vi "ExperimentCode_nodaq.vi"() -> ()   [LabVIEW 2017]
uses:
  <vilib>/Analysis/baseanly.llb/Mean (DBL).vi
  <vilib>/Instr/_visa.llb/VISA Configure Serial Port (Instr).vi
  <vilib>/express/express shared/transition.llb/Dynamic To Waveform Array.vi
  <vilib>/express/express signal manip/GetorSetDDTAttributes/Set DDT Attributes/SetT0.vi
  <vilib>/express/express shared/transition.llb/Waveform Array To Dynamic.vi
  <vilib>/express/express signal manip/GetorSetDDTAttributes/Set DDT Attributes/Set DDT Properties.xnode
  <vilib>/Analysis/NI_AALPro.lvlib
  <vilib>/Analysis/NI_AALBase.lvlib
panel:
  in  "Tab Control":enum32{"Setup ", "Experiment Controls", "Debug"}(tab)=enum."Experiment Controls"
  in  "Axial Force Slope":dbl=1.0
  in  "Axial Force Intercept":dbl
  in  "Side Force Slope":dbl=1.0
  in  "Side Force Intercept":dbl
  in  "Yaw Moment Slope":dbl=1.0
  in  "Yaw Moment Intercept":dbl
  in  "Max Torque":dbl=21.3
  in  "Servo 1 Zero Offset":dbl
  in  "Servo 2 Zero Offset":dbl
  in  "Servo 3 Zero Offset":dbl
  in  "Servo 4 Zero Offset":dbl
  in  "Servo 5 Zero Offset":dbl
  in  "Servo 5 Torque Intercept":dbl
  in  "Servo 5 Torque Slope":dbl=1.0
  in  "Servo 5 Position Intercept":dbl
  in  "Servo 5 Position Slope":dbl=1.0
  in  "Servo 4 Torque Intercept":dbl
  in  "Servo 4 Torque Slope":dbl=1.0
  in  "Servo 4 Position Intercept":dbl
  in  "Servo 4 Position Slope":dbl=1.0
  in  "Servo 3 Torque Intercept":dbl
  in  "Servo 3 Torque Slope":dbl=1.0
  in  "Servo 3 Position Intercept":dbl=-111.82
  in  "Servo 3 Position Slope":dbl=0.00449
  in  "Servo 2 Torque Intercept":dbl
  in  "Servo 2 Torque Slope":dbl=1.0
  in  "Servo 2 Position Intercept":dbl=-97.9723
  in  "Servo 2 Position Slope":dbl=0.00488
  in  "Servo 1 Torque Intercept":dbl
  in  "Servo 1 Torque Slope":dbl=1.0
  in  "Servo 1 Position Intercept":dbl=-99.625
  in  "Servo 1 Position Slope":dbl=0.004988
  in  "Plot Last x Seconds":dbl=60.0
  in  "COM Port":refnum<visa-resource-name>
  in  "Buad Rate":i32(ring)=115200 items=["2400"=2400, "4800"=4800, "9600"=9600, "14400"=14400, "19200"=19200, "28800"=28800, "38400"=38400, "57600"=57600, "115200"=115200]
  in  "Lowest Servo Angle":dbl=-65.0
  in  "Highest Servo Angle":dbl=65.0
  in  "Number of Servos":dbl=5.0
  out "Lift FFT":cluster{"timeout (s)":dbl, dbl, dbl[]}(graph)={"timeout (s)"=0.0, 0.12149192078726764, [0.041647829769514415, 0.5815679381268424, 0.2410963163674246, 0.13249316216492138, 0.09139863383267581, 0.06777994108166811, 0.05676278057361634, 0.046891488943555756, 0.04170299677912171, 0.03813645823405653, 0.032751623310567676, 0.03235242616779546, 0.02857646287326414, 0.027921332836055062, 0.026075669248962027, 0.025506839186418245, 0.02300088021285802, 0.022263519164960176, 0.020785068115577936, 0.020572576904436635, 0.019706083690027066, 0.01933094658327721, 0.018088168860478246, 0.018107278585544298, 0.016955162903130913, 0.016878745360566313, 0.015869739803903514, 0.015674152094024396, 0.016464851454026343, 0.015714406087046065, 0.015341040986334412, 0.015154899432712336, 0.014786629089704205, 0.01448548753300844, 0.014186097789199267, 0.014076976739574329, 0.013620814630327938, 0.014015320026164364, 0.013807357325215744, 0.01339057225347958, 0.01298234875346484, 0.013354575711390817, 0.013214518458269849, 0.013075613311439785, 0.012989188265392547, 0.012875952831802175]}
  out "Maximum Torque Exceeded":bool
  in  "Amplitude (deg)":dbl=3.0
  in  "Save":bool
  in  "Stop VI":bool
  in  "Sample Frequency":dbl=100.0 step=50.0
  out "Servo Torque":cluster{" Time Offset":dbl, dbl, dbl[][]}(graph)
  in  "Amplitude (cm)":dbl=4.0
  in  "Length of Segments":dbl=10.0
  in  "Number of Waves":dbl=1.0
  in  "Wave Exponential":dbl=2.0
  in  "Frequency":dbl=1.0
  in  "Wave Form":u16(ring) items=["Sine", "Exponentional Sine", "Second Mode Bending", "Flat Plate"]
  in  "Wind Up Waveform":bool
  in  "Mode 1 Amplitude":dbl=0.1 step=0.1
  in  "Mode 2 Amplitude":dbl=0.2 step=0.1
  in  "Mode 1 Phase":dbl step=0.1
  in  "Mode 2 Phase":dbl=0.8499 step=0.1
  in  "Wind Down Waveform":bool
  in  "Wind Down Time":i32=5
  out "Waveform":cluster{"X Nodes":dbl[], "Y Nodes":dbl[]}[](graph)
  in  "Servo Input":bool
  in  "Send To Waveform to MBE":bool
  in  "Servo 5 Input":dbl
  in  "Servo 4 Input":dbl
  in  "Servo 3 Input":dbl
  in  "Servo 2 Input":dbl
  in  "Servo 1  Input":dbl
  out "Force and Moment Data":cluster{" Time Offset":dbl, "mean":dbl, dbl[][]}(graph)
  out "Minimum or Maximum Angle Exceeded":bool
  in  "Filename":path=path "test.tdms"
  out "Drag FFT":cluster{"timeout (s)":dbl, dbl, dbl[]}(graph)={"timeout (s)"=0.0, 0.12149192078726764, [0.08329565953902883, 1.1631358762536848, 0.4821926327348492, 0.26498632432984276, 0.18279726766535162, 0.13555988216333623, 0.11352556114723268, 0.09378297788711151, 0.08340599355824342, 0.07627291646811306, 0.06550324662113535, 0.06470485233559092, 0.05715292574652828, 0.055842665672110124, 0.052151338497924055, 0.05101367837283649, 0.04600176042571604, 0.04452703832992035, 0.04157013623115587, 0.04114515380887327, 0.03941216738005413, 0.03866189316655442, 0.03617633772095649, 0.036214557171088596, 0.033910325806261826, 0.03375749072113263, 0.03173947960780703, 0.03134830418804879, 0.03292970290805269, 0.03142881217409213, 0.030682081972668824, 0.030309798865424672, 0.02957325817940841, 0.02897097506601688, 0.028372195578398533, 0.028153953479148657, 0.027241629260655875, 0.028030640052328727, 0.02761471465043149, 0.02678114450695916, 0.02596469750692968, 0.026709151422781633, 0.026429036916539698, 0.02615122662287957, 0.025978376530785094, 0.02575190566360435]}
  in  "Comment":string
  out "Yaw FFT":cluster{"timeout (s)":dbl, dbl, dbl[]}(graph)={"timeout (s)"=0.0, 0.12149192078726764, [0.004164782976951441, 0.05815679381268424, 0.024109631636742457, 0.013249316216492139, 0.009139863383267582, 0.006777994108166813, 0.005676278057361634, 0.004689148894355577, 0.0041702996779121706, 0.0038136458234056527, 0.0032751623310567674, 0.0032352426167795464, 0.0028576462873264145, 0.0027921332836055067, 0.0026075669248962034, 0.002550683918641824, 0.002300088021285804, 0.002226351916496017, 0.0020785068115577923, 0.0020572576904436613, 0.0019706083690027043, 0.0019330946583277187, 0.0018088168860478228, 0.001810727858554431, 0.0016955162903130908, 0.0016878745360566349, 0.001586973980390353, 0.0015674152094024417, 0.001646485145402633, 0.0015714406087046053, 0.00153410409863344, 0.0015154899432712331, 0.0014786629089704193, 0.001448548753300844, 0.001418609778919927, 0.0014076976739574325, 0.0013620814630327948, 0.0014015320026164368, 0.0013807357325215724, 0.0013390572253479574, 0.0012982348753464844, 0.001335457571139084, 0.0013214518458269826, 0.0013075613311439762, 0.0012989188265392561, 0.0012875952831802166]}
  out "Specified Time Delay":dbl
  out "Calculated Time Delay":dbl
  out "Time Elapsed":dbl
  out "Output Angles":dbl[](array[numeric])
  out "Input Angles":dbl[](array[numeric])
  out "Pos5 number":dbl
  out "Pos4 number":dbl
  out "Pos3 number":dbl
  out "Pos2 number":dbl
  out "Pos1 number":dbl
  out "Torq1 number":dbl
  out "Torq2 number":dbl
  out "Torq3 number":dbl
  out "Torq4 number":dbl
  out "Torq5 number":dbl
  out "Servo 1 Position":cluster{" Time Offset":dbl, "mean":dbl, dbl[][]}(graph)
  out "Servo 2 Position":cluster{" Time Offset":dbl, "mean":dbl, dbl[][]}(graph)
  out "Servo 3 Position":cluster{" Time Offset":dbl, "mean":dbl, dbl[][]}(graph)
  out "Servo 4 Position":cluster{" Time Offset":dbl, "mean":dbl, dbl[][]}(graph)
  out "Servo 5 Position":cluster{" Time Offset":dbl, "mean":dbl, dbl[][]}(graph)
  out "Sent to Arduino":string
  out "Bytes at port":cluster{i32, dbl, dbl[]}(graph)
  out "Read Buffer":string
  out "X Nodes":dbl[](array[numeric])
  out "Y Nodes":dbl[](array[numeric])
  # "deg"
  # "deg"
  # "deg"
  # "deg"
  # "deg"
  # "Waveform"
  # "Manual"
  # "cm"
  # "Hz"
  # "Off"
  # "On"
  # "rad"
  # "rad"
  # "Off"
  # "On"
  # "Hz"
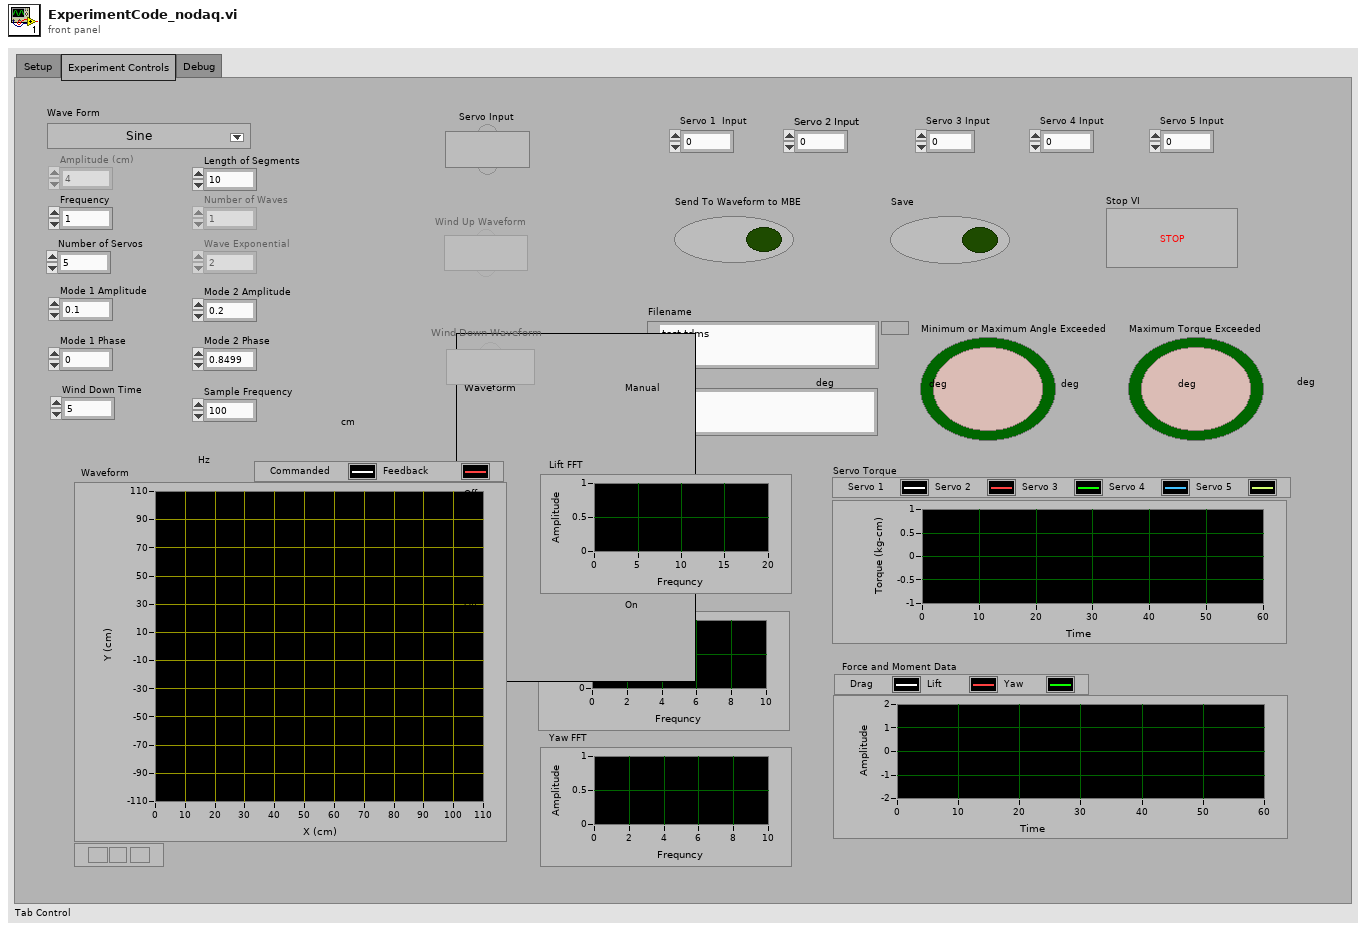
[diagram p1: front panel]
types:
  T1 = enum8{"Enabled", "Disabled", "Disabled and Grayed Out"}
  T2 = cluster{"Amplitude (deg)":dbl, "Amplitude (cm)":dbl, "Frequency":dbl, "Number of Waves":dbl, "Length of Segments":dbl, "Wave Exponential":dbl, "Number of Servos":dbl, "Mode 1 Amplitude":dbl, "Mode 2 Amplitude":dbl, "Mode 1 Phase":dbl, "Mode 2 Phase":dbl}
  T3 = cluster{"timeout (s)":dbl, "df":dbl, "Amp Spectrum Mag (Vrms)":dbl[]}
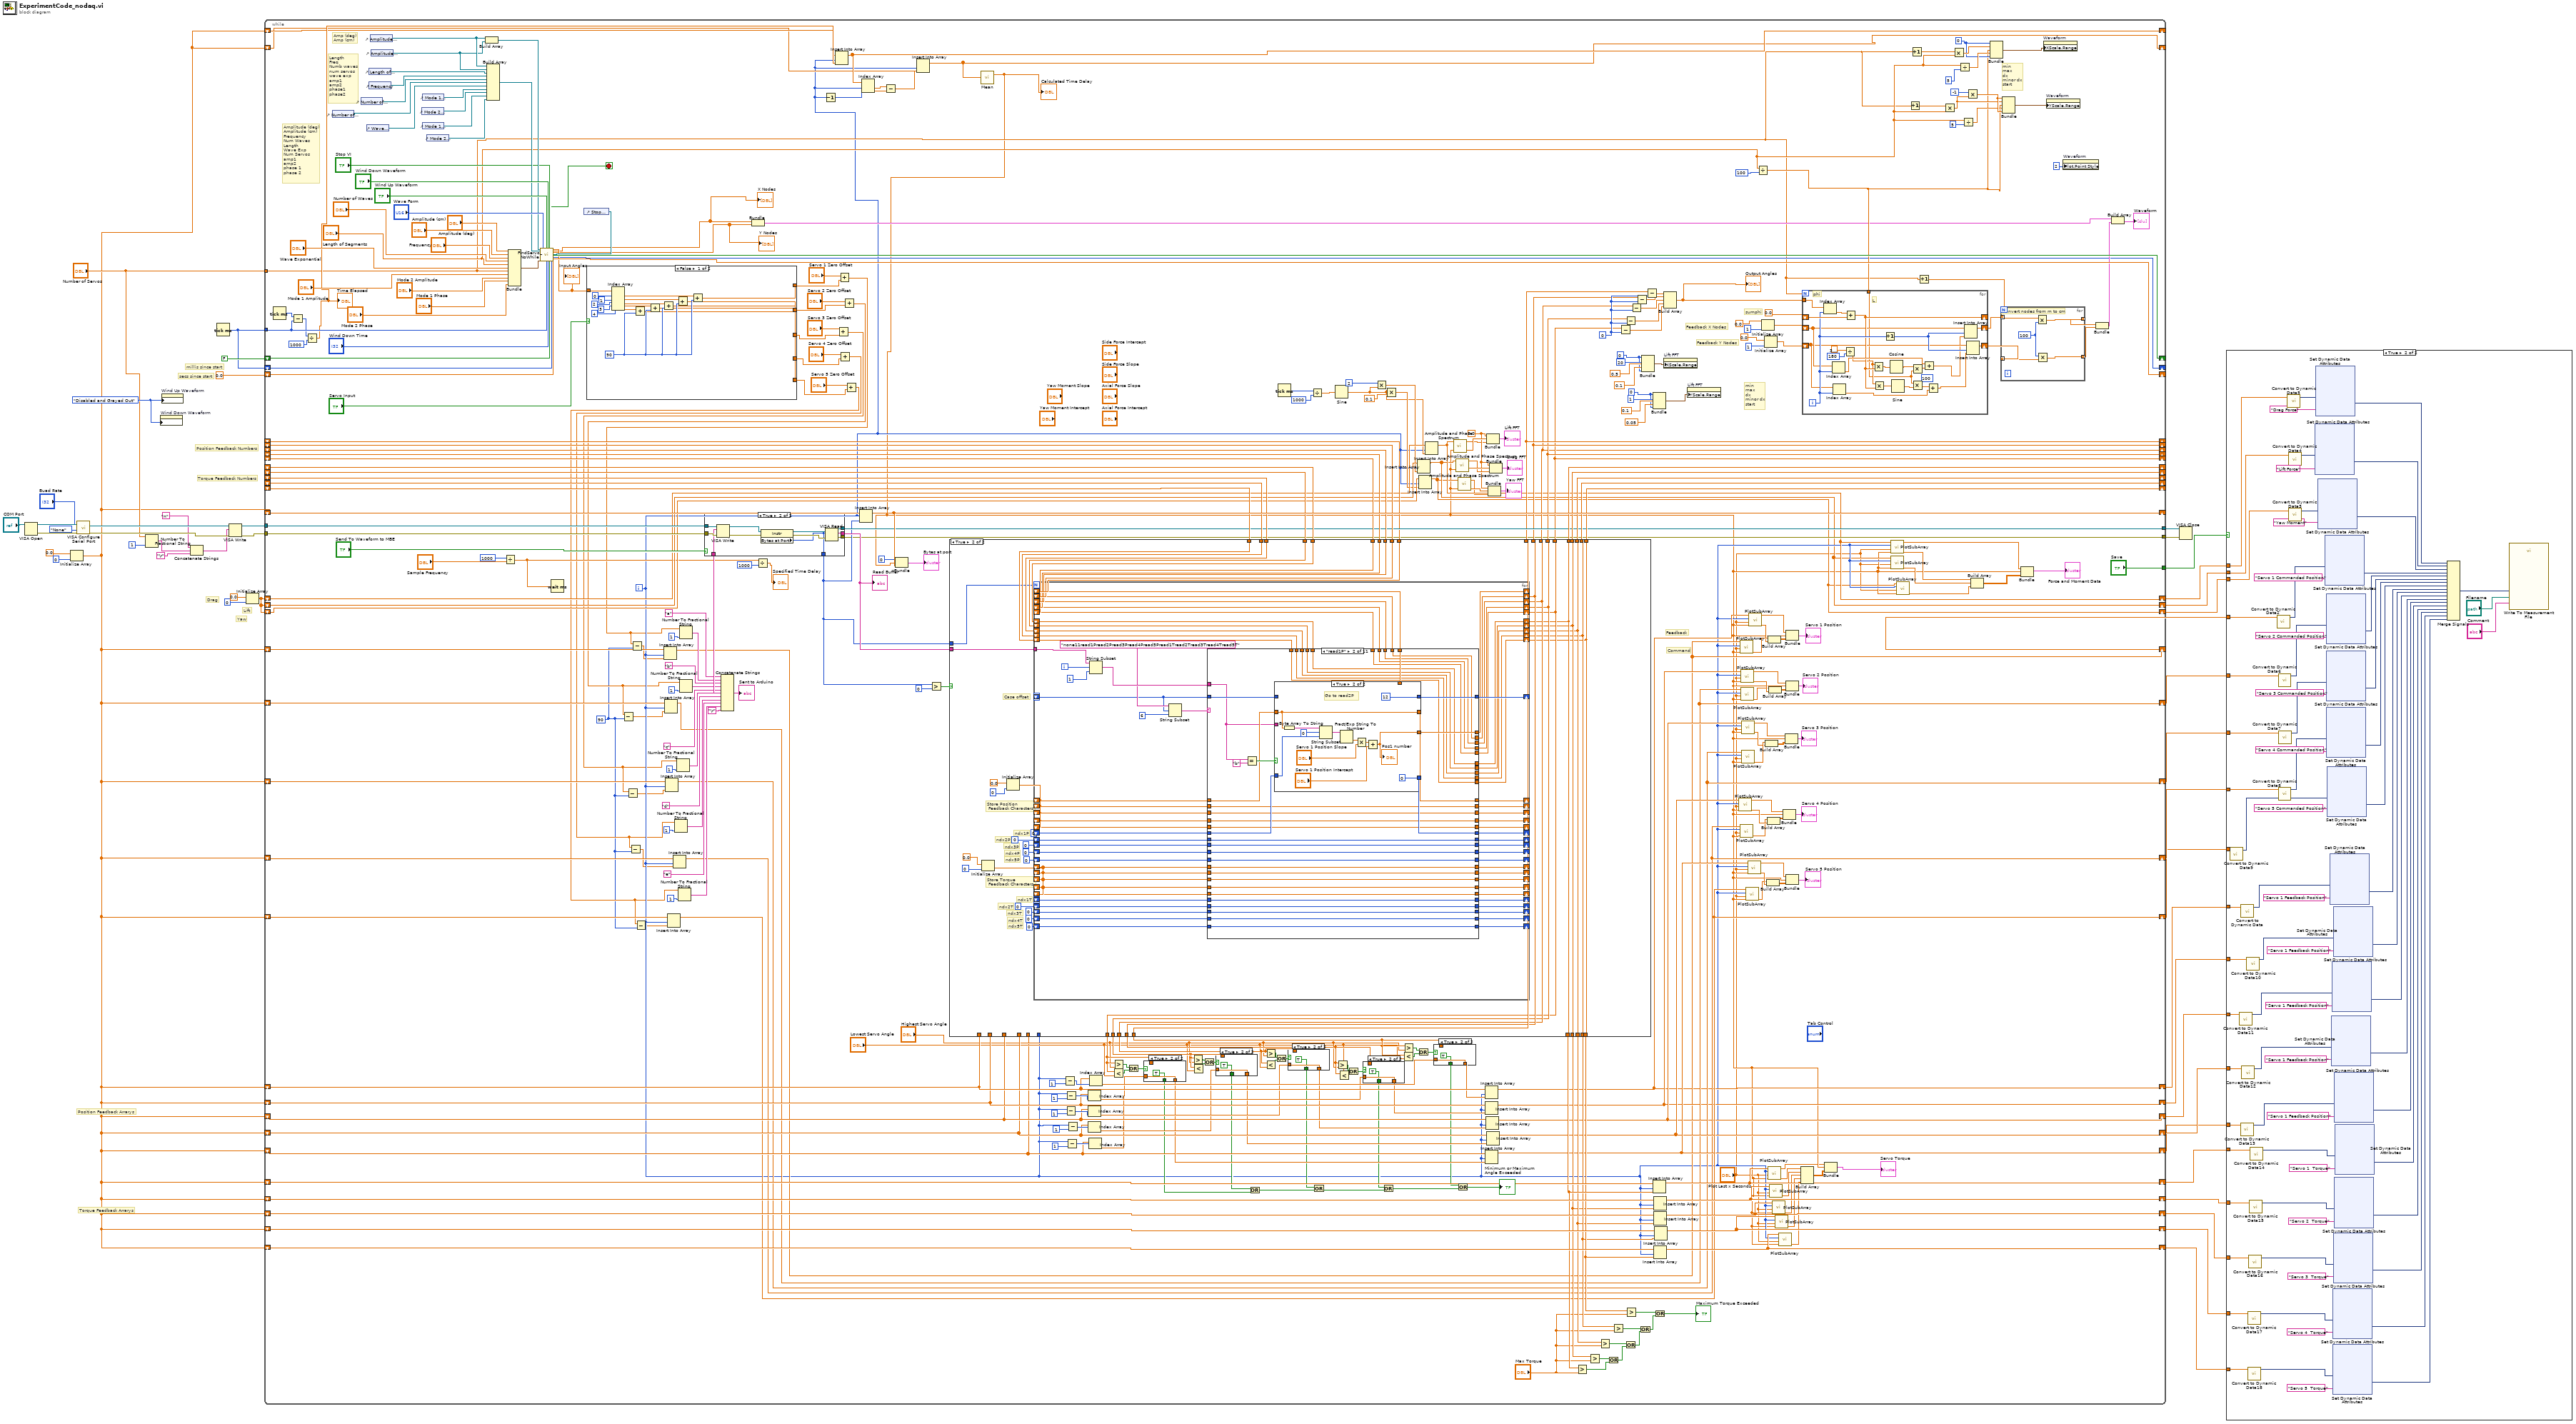
[diagram p0: block diagram]
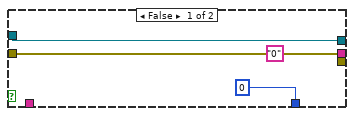
[diagram p3: hidden frame]
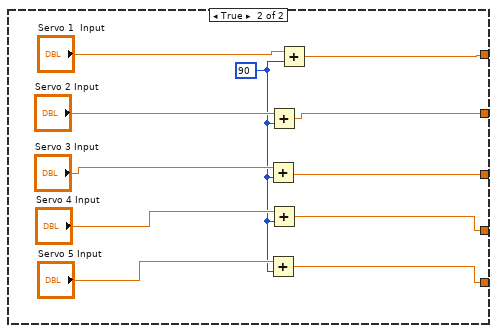
[diagram p4: hidden frame]
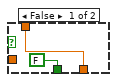
[diagram p5: hidden frame]
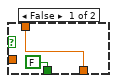
[diagram p6: hidden frame]
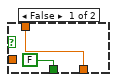
[diagram p7: hidden frame]
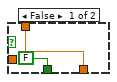
[diagram p8: hidden frame]
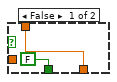
[diagram p9: hidden frame]
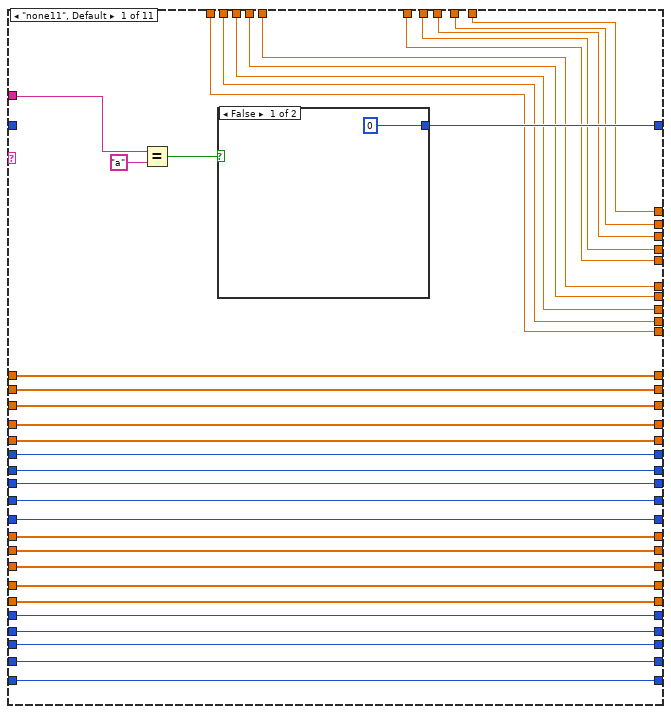
[diagram p11: hidden frame]
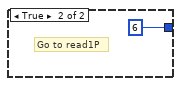
[diagram p12: hidden frame]
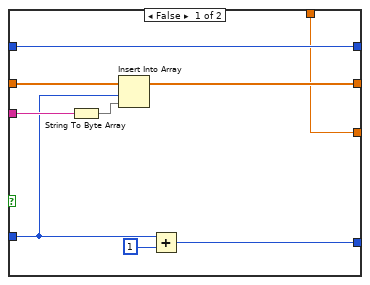
[diagram p13: hidden frame]
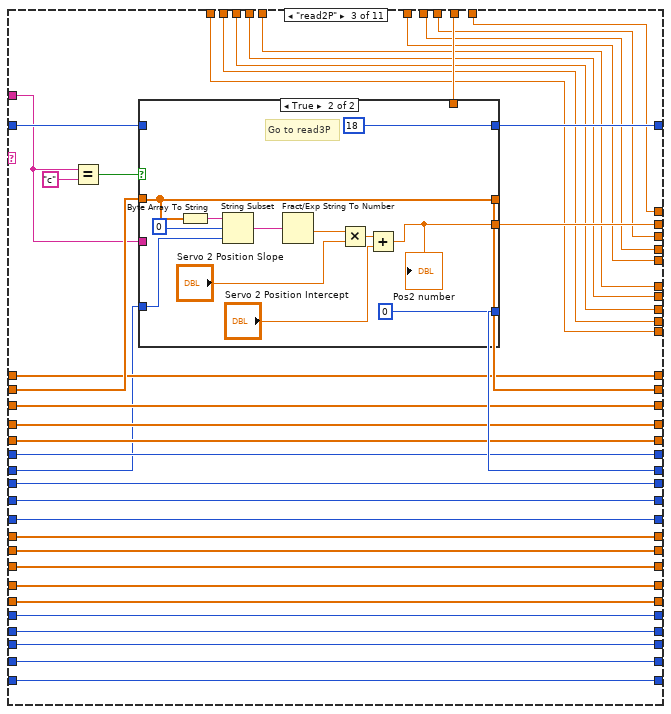
[diagram p14: hidden frame]
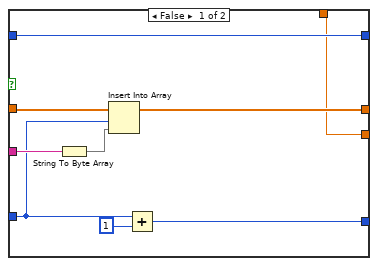
[diagram p15: hidden frame]
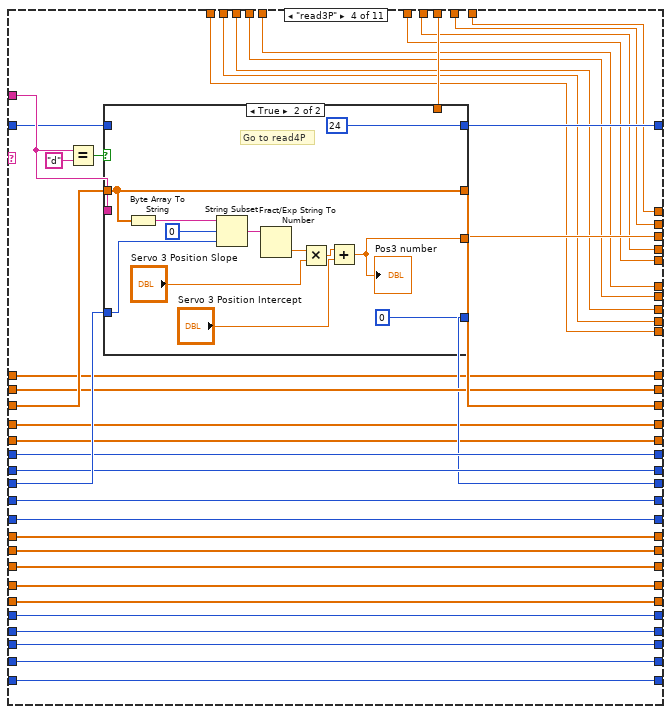
[diagram p16: hidden frame]
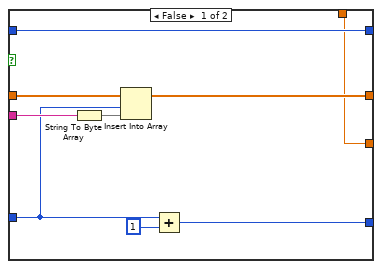
[diagram p17: hidden frame]
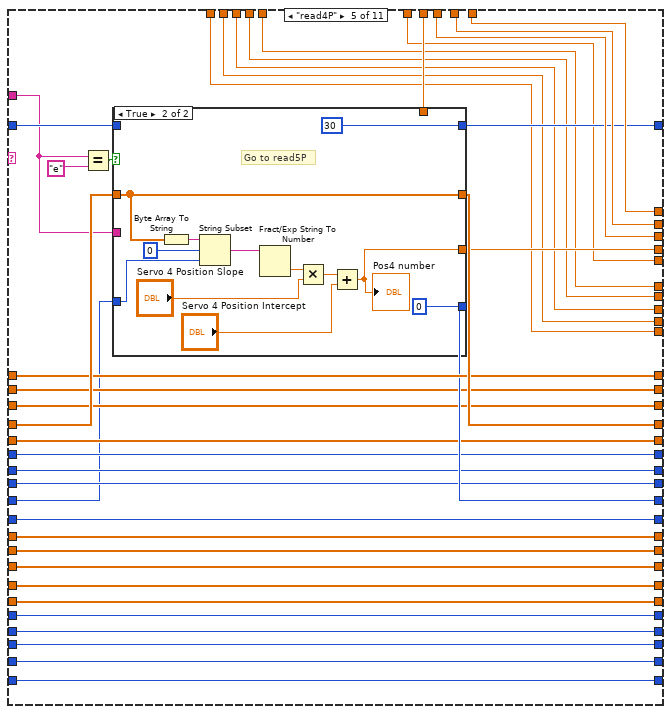
[diagram p18: hidden frame]
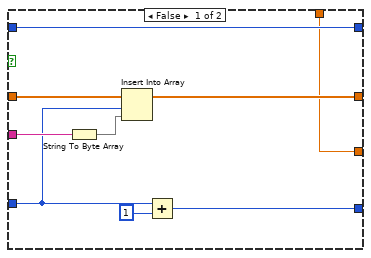
[diagram p19: hidden frame]
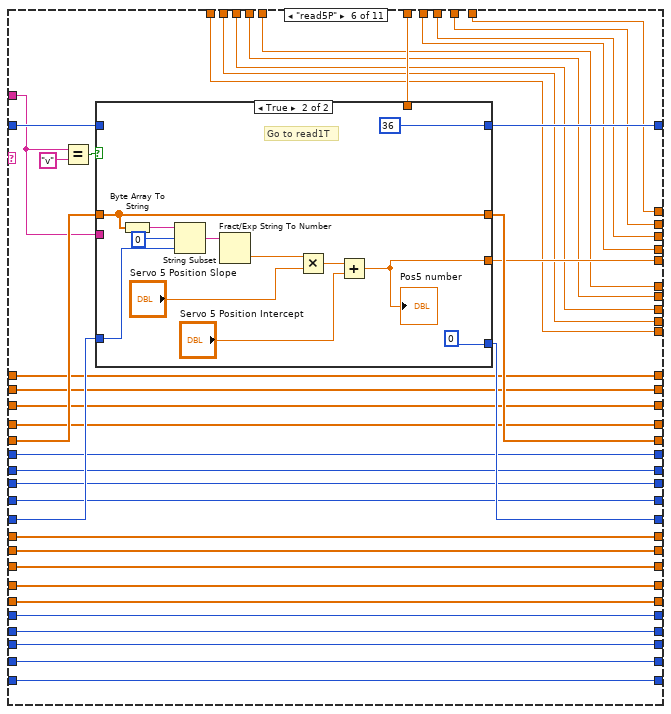
[diagram p20: hidden frame]
diagram:
  w28 = T1."Disabled and Grayed Out" ("Disabled")
  # "Yaw"
  # "Lift"
  # "secs since start"
  # "millis since start"
  # "Drag"
  # "Torque Feedback Numbers"
  # "Position Feedback Numbers"
  # "Torque Feedback Arrarys"
  # "Position Feedback Arrarys"
  n1 = VISA Open(VISA resource name="COM Port") -> (VISA resource name=w43:refnum<visa-resource-name>, error out=w41:errorcluster)  [unwired: 4 in]
  n2 = Initialize Array(0.0 ("element"), 0 ("dimension size")) -> (w1:dbl[])
  n3 = call-poly "VISA Configure Serial Port"("VISA resource name"=w43, "baud rate (9600)"="Buad Rate", "parity (0:none)"=enum16{"None", "Odd", "Even", "Mark", "Space"}."None", "error in (no error)"=w41) -> ("VISA resource name out"=w11:refnum<visa-resource-name>, "error out"=w10:errorcluster)  [unwired: 10 in]
  n4 = Number To Fractional String(number="Number of Servos", precision (6)=1) -> (F-format string=w6:string)  [unwired: 2 in]
  n5 = property on="Wind Down Waveform" class="Bool (strict)"("DisabledEnum"=w28) -> ()  [unwired: 2 in, 2 out]
  n6 = property on="Wind Up Waveform" class="Bool (strict)"("DisabledEnum"=w28) -> ()  [unwired: 2 in, 2 out]
  n7 = Concatenate Strings("n", w6, "\r") -> (w2:string)
  n8 = Tick Count (ms)() -> (millisecond timer value=w37:u32)
  n9 = VISA Write(VISA resource name=w11, write buffer=w2, error in (no error)=w10) -> (VISA resource name out=w9:refnum<visa-resource-name>, error out=w8:errorcluster)  [unwired: 1 out]
  n10 = Initialize Array(0.0 ("element"), 0 ("dimension size")) -> (w29:dbl[])
  n11 = while {
    shift-right: [w387] -> _
    shift-left: w1 -> [w388]
    shift-right: [w93] -> w35
    shift-left: w1 -> [w364]
    shift-right: [w95] -> w24
    shift-left: w1 -> [w363]
    shift-right: [w99] -> w23
    shift-left: w1 -> [w362]
    shift-right: [w101] -> w22
    shift-left: w1 -> [w361]
    shift-right: [w109] -> w21
    shift-left: w1 -> [w360]
    shift-right: [w92] -> w31
    shift-left: w1 -> [w328]
    shift-right: [w94] -> w20
    shift-left: w1 -> [w320]
    shift-right: [w98] -> w19
    shift-left: w1 -> [w317]
    shift-right: [w102] -> w18
    shift-left: w1 -> [w314]
    shift-right: [w108] -> w17
    shift-left: w1 -> [w284]
    shift-right: [w185] -> _
    shift-left: _ -> [w331]
    shift-right: [w184] -> _
    shift-left: _ -> [w350]
    shift-right: [w181] -> _
    shift-left: _ -> [w353]
    shift-right: [w183] -> _
    shift-left: _ -> [w352]
    shift-right: [w182] -> _
    shift-left: _ -> [w351]
    shift-right: [w344] -> _
    shift-left: _ -> [w345]
    shift-right: [w343] -> _
    shift-left: _ -> [w346]
    shift-right: [w342] -> _
    shift-left: _ -> [w347]
    shift-right: [w341] -> _
    shift-left: _ -> [w348]
    shift-right: [w340] -> _
    shift-left: _ -> [w349]
    shift-right: [w226] -> w16
    shift-left: w1 -> [w339]
    shift-right: [w224] -> w15
    shift-left: w1 -> [w338]
    shift-right: [w223] -> w14
    shift-left: w1 -> [w337]
    shift-right: [w222] -> w13
    shift-left: w1 -> [w336]
    shift-right: [w225] -> w12
    shift-left: w1 -> [w335]
    tunnel: w8 -> [w283]
    shift-right: [w89] -> w27
    shift-left: w29 -> [w147]
    tunnel: w37 -> [w126]
    shift-right: [w277] -> _
    shift-left: FALSE -> [w274]
    shift-right: [w116] -> _
    shift-left: w37 -> [w122]
    shift-right: [w276] -> _
    shift-left: 0.0 ("S since stop Shift Out") -> [w123]
    tunnel: ["Save"] -> w34
    tunnel: w9 -> [w282]
    tunnel: [w332] -> w33
    tunnel: [w154] -> w32
    shift-right: [w73] -> w26
    shift-left: w29 -> [w146]
    shift-right: [w72] -> w25
    shift-left: w29 -> [w145]
    shift-right: [w113] -> _
    shift-left: w1 -> [w120]
    tunnel: "Number of Servos" -> [w115]
    shift-right: [w110] -> _
    shift-left: w1 -> [w111]
    i -> [w84]
    stop <- w236 stop-if-true
    w49 = 90
    w132 = 0
    w136 = 0
    w65 = 0.0 ("timeout (s)")
    w170 = 0
    w186 = 0
    # "min\nmax\ndx\nminor dx\nstart"
    # "min\nmax\ndx\nminor dx\nstart"
    # "Feedback Y Nodes"
    # "Feedback X Nodes"
    # "sumphi"
    # "Command"
    # "Feedback"
    # "Amplitude (deg)\nAmplitude (cm)\nFrequency\nNum Waves\nLength\nWave Exp\nNum Servos\namp1\namp2\nphase 1\nphase 2"
    # "Amp (deg)\nAmp (cm)"
    # "Length\nFreq\nNumb waves\nnum servos\nwave exp\namp1\namp2\nphase1\nphase2"
    n12 = Tick Count (ms)() -> (millisecond timer value=w127:u32)
    n13 = Subtract(x=w127, y=w126) -> (x-y=w125:u32)
    n14 = Divide(x=w125, y=1000) -> (x/y=w121:dbl)
    "Time Elapsed" <- w121
    n15 = control-ref of="Number of Servos"() -> (w114:refnum<vi>)
    n16 = control-ref of="Number of Waves"() -> (w259:refnum<vi>)
    n17 = control-ref of="Wave Exponential"() -> (w258:refnum<vi>)
    n18 = control-ref of="Length of Segments"() -> (w261:refnum<vi>)
    n19 = control-ref of="Frequency"() -> (w260:refnum<vi>)
    n20 = control-ref of="Amplitude (deg)"() -> (w241:refnum<vi>)
    n21 = control-ref of="Amplitude (cm)"() -> (w240:refnum<vi>)
    n22 = control-ref of="Mode 2 Amplitude"() -> (w256:refnum<vi>)
    n23 = control-ref of="Mode 1 Amplitude"() -> (w257:refnum<vi>)
    n24 = control-ref of="Mode 1 Phase"() -> (w255:refnum<vi>)
    n25 = control-ref of="Mode 2 Phase"() -> (w254:refnum<vi>)
    n26 = Build Array(w241, w240) -> (w243:refnum<vi>[])
    n27 = Build Array(w241, w240, w261, w260, w259, w114, w258, w257, w256, w255, w254) -> (w242:refnum<vi>[])
    n28 = Divide(x=1000, y="Sample Frequency") -> (x/y=w129:dbl)
    n29 = Bundle("Amplitude (deg)"="Amplitude (deg)", "Amplitude (cm)"="Amplitude (cm)", "Frequency"="Frequency", "Number of Waves"="Number of Waves", "Length of Segments"="Length of Segments", "Wave Exponential"="Wave Exponential", "Number of Servos"=w115, "Mode 1 Amplitude"="Mode 1 Amplitude", "Mode 2 Amplitude"="Mode 2 Amplitude", "Mode 1 Phase"="Mode 1 Phase", "Mode 2 Phase"="Mode 2 Phase") -> (w244:T2)  [unwired: 1 in]
    n30 = Wait (ms)(milliseconds to wait=w129) -> ()  [unwired: 1 out]
    n31 = control-ref of="Stop Reference"() -> (w273:refnum<vi>)
    n32 = call "FindServo_NoWhile.vi"("Amplitude Reference Array"=w243, "Parameter Reference Arrary"=w242, "Parameter Cluster"=w244, "Wave Form"="Wave Form", "Wind Up"="Wind Up Waveform", "Start Time (Tick Count-millis)"=w126, "Wind Down"="Wind Down Waveform", "Wind Down Time"="Wind Down Time", "Stop In"="Stop VI", "Stop Pressed Shift In (False)"=w274, "Ms Since Stop Shift In (Start Time)"=w122, "Stop In Reference"=w273, "S since stop Shift In"=w123) -> ("Stop Out"=w236:bool, "phi"=w155:dbl[], "X Nodes"=w48:dbl[], "Y Nodes"=w47:dbl[], "Stop Pressed Shift Out (False)"=w277:bool, "MS Since Stop Shift Out"=w116:u32, "S since stop Shift Out"=w276:dbl)  [unwired: 8 in]
    "Input Angles" <- w155
    "X Nodes" <- w48
    "Y Nodes" <- w47
    n33 = case shown="False" "Servo Input" {
      tunnel: [w437 w460] -> w267
      tunnel: [w436 w452] -> w266
      tunnel: [w435 w451] -> w265
      tunnel: [w434 w456] -> w264
      tunnel: [w433 w457] -> w263
      tunnel: w155 -> [w449 _]
      frame False {
        w438 = 90
        n34 = Index Array(array=w449, index #1=0, index #2=1, index #3=2, index #4=3, index #5=4) -> (element #1=w443:dbl, element #2=w442:dbl, element #3=w441:dbl, element #4=w440:dbl, element #5=w439:dbl)
        n35 = Add(x=w439, y=w438) -> (x+y=w433:dbl)
        n36 = Add(x=w440, y=w438) -> (x+y=w434:dbl)
        n37 = Add(x=w441, y=w438) -> (x+y=w435:dbl)
        n38 = Add(x=w442, y=w438) -> (x+y=w436:dbl)
        n39 = Add(x=w443, y=w438) -> (x+y=w437:dbl)
      }
      frame True {
        w450 = 90
        n40 = Add(x="Servo 3 Input", y=w450) -> (x+y=w451:dbl)
        n41 = Add(x="Servo 5 Input", y=w450) -> (x+y=w457:dbl)
        n42 = Add(x="Servo 2 Input", y=w450) -> (x+y=w452:dbl)
        n43 = Add(x="Servo 4 Input", y=w450) -> (x+y=w456:dbl)
        n44 = Add(x="Servo 1  Input", y=w450) -> (x+y=w460:dbl)
      }
    }
    n45 = Bundle("X Nodes"=w48, "Y Nodes"=w47) -> (w165:cluster{"X Nodes":dbl[], "Y Nodes":dbl[]})  [unwired: 1 in]
    n46 = Divide(x=w129, y=1000) -> (x/y=→"Specified Time Delay":dbl)
    n47 = Decrement(x=w84) -> (x-1=w117:i32)
    n48 = Insert Into Array(array=w120, index=w84, new element=w121) -> (w113:dbl[])
    n49 = Add(x="Servo 3 Zero Offset", y=w265) -> (x+y=w54:dbl)
    n50 = Subtract(x=w54, y=w49) -> (x-y=w55:dbl)
    n51 = Insert Into Array(array=w362, index=w84, new element=w55) -> (w99:dbl[])
    n52 = Number To Fractional String(number=w54, precision (6)=1) -> (F-format string=w383:string)  [unwired: 2 in]
    n53 = Add(x="Servo 1 Zero Offset", y=w267) -> (x+y=w58:dbl)
    n54 = Subtract(x=w58, y=w49) -> (x-y=w59:dbl)
    n55 = Insert Into Array(array=w364, index=w84, new element=w59) -> (w93:dbl[])
    n56 = Number To Fractional String(number=w58, precision (6)=1) -> (F-format string=w385:string)  [unwired: 2 in]
    n57 = Add(x="Servo 4 Zero Offset", y=w264) -> (x+y=w52:dbl)
    n58 = Subtract(x=w52, y=w49) -> (x-y=w53:dbl)
    n59 = Insert Into Array(array=w361, index=w84, new element=w53) -> (w101:dbl[])
    n60 = Number To Fractional String(number=w52, precision (6)=1) -> (F-format string=w376:string)  [unwired: 2 in]
    n61 = Add(x="Servo 2 Zero Offset", y=w266) -> (x+y=w56:dbl)
    n62 = Subtract(x=w56, y=w49) -> (x-y=w57:dbl)
    n63 = Insert Into Array(array=w363, index=w84, new element=w57) -> (w95:dbl[])
    n64 = Number To Fractional String(number=w56, precision (6)=1) -> (F-format string=w384:string)  [unwired: 2 in]
    n65 = Add(x="Servo 5 Zero Offset", y=w263) -> (x+y=w50:dbl)
    n66 = Subtract(x=w50, y=w49) -> (x-y=w51:dbl)
    n67 = Insert Into Array(array=w360, index=w84, new element=w51) -> (w109:dbl[])
    n68 = Number To Fractional String(number=w50, precision (6)=1) -> (F-format string=w375:string)  [unwired: 2 in]
    n69 = Concatenate Strings("a", w385, "b", w384, "c", w383, "d", w376, "e", w375, "\r") -> (w386:string)
    "Sent to Arduino" <- w386
    n70 = case shown="True" "Send To Waveform to MBE" {
      tunnel: w386 -> [_ w422]
      tunnel: ["0" w432] -> w371
      tunnel: [w420 w431] -> w154
      tunnel: [w421 w430] -> w332
      tunnel: [0 w425] -> w239
      tunnel: w283 -> [w420 w424]
      tunnel: w282 -> [w421 w423]
      frame False {
      }
      frame True {
        n71 = VISA Write(VISA resource name=w423, write buffer=w422, error in (no error)=w424) -> (VISA resource name out=w429:refnum<visa-resource-name>, error out=w426:errorcluster)  [unwired: 1 out]
        n72 = property class="Instr"(reference=w429, error in=w426) -> (reference out=w428:refnum<visa-resource-name>, error out=w427:errorcluster, "Bytes at Port"=w425:u32)
        n73 = VISA Read(VISA resource name=w428, byte count=w425, error in (no error)=w427) -> (VISA resource name out=w430:refnum<visa-resource-name>, read buffer=w432:string, error out=w431:errorcluster)  [unwired: 1 out]
      }
    }
    "Read Buffer" <- w371
    n74 = Insert Into Array(array=w388, index=w84, new element=w239) -> (w387:dbl[])
    n75 = Index Array(array=w113, index #1=w84, index #2=w117) -> (element #1=w119:dbl, element #2=w118:dbl)
    n76 = Subtract(x=w119, y=w118) -> (x-y=w112:dbl)
    n77 = Insert Into Array(array=w111, index=w84, new element=w112) -> (w110:dbl[])
    n78 = Greater?(x=w239, y=0) -> (0:w334:bool)
    n79 = case shown="True" w334 {
      tunnel: w239 -> [_ w491]
      tunnel: w371 -> [_ w529]
      tunnel: [w490 w503] -> w323
      tunnel: w84 -> [_ _]
      tunnel: w328 -> [_ _]
      tunnel: [w489 w502] -> w305
      tunnel: [w488 w501] -> w299
      tunnel: [w487 w500] -> w293
      tunnel: [w486 w499] -> w289
      tunnel: w320 -> [_ _]
      tunnel: w317 -> [_ _]
      tunnel: w314 -> [_ _]
      tunnel: w284 -> [_ _]
      tunnel: w331 -> [w490 w520]
      tunnel: w350 -> [w489 w519]
      tunnel: w353 -> [w488 w518]
      tunnel: w352 -> [w487 w517]
      tunnel: w351 -> [w486 w516]
      tunnel: [w490 w503] -> w185
      tunnel: [w489 w502] -> w184
      tunnel: [w488 w501] -> w181
      tunnel: [w487 w500] -> w183
      tunnel: [w486 w499] -> w182
      tunnel: w349 -> [w481 w493]
      tunnel: w348 -> [w482 w495]
      tunnel: w347 -> [w483 w515]
      tunnel: w346 -> [w484 w514]
      tunnel: w345 -> [w485 w513]
      tunnel: [w485 w498] -> w344
      tunnel: [w484 w497] -> w343
      tunnel: [w483 w496] -> w342
      tunnel: [w482 w494] -> w341
      tunnel: [w481 w492] -> w340
      tunnel: [w485 w498] -> w214
      tunnel: [w484 w497] -> w210
      tunnel: [w483 w496] -> w211
      tunnel: [w482 w494] -> w212
      tunnel: [w481 w492] -> w213
      frame False {
      }
      frame True {
        # "Store Torque\n Feedback Characters"
        # "ndx5T"
        # "ndx4T"
        # "ndx3T"
        # "ndx2T"
        # "ndx1T"
        # "Store Position\n Feedback Characters"
        # "ndx5P"
        # "ndx4P"
        # "ndx3P"
        # "ndx2P"
        # "ndx1P"
        # "Case offset"
        n80 = Initialize Array(0.0 ("element"), 0 ("dimension size")) -> (w510:dbl[])
        n81 = Initialize Array(0.0 ("element"), 0 ("dimension size")) -> (w523:dbl[])
        n82 = for {
          N: w491 -> [_]
          tunnel: w529 -> [w597]
          shift-right: [w595] -> _
          shift-left: 1 -> [w540]
          shift-right: [w594] -> _
          shift-left: 0 -> [w593]
          shift-right: [w591] -> _
          shift-left: w523 -> [w592]
          shift-right: [w589] -> _
          shift-left: w523 -> [w590]
          shift-right: [w585] -> _
          shift-left: 0 -> [w588]
          shift-right: [w586] -> _
          shift-left: 0 -> [w587]
          shift-right: [w583] -> _
          shift-left: w523 -> [w584]
          shift-right: [w575] -> _
          shift-left: w523 -> [w582]
          shift-right: [w576] -> _
          shift-left: w523 -> [w581]
          shift-right: [w579] -> _
          shift-left: 0 -> [w580]
          shift-right: [w577] -> _
          shift-left: 0 -> [w578]
          shift-right: [w562] -> _
          shift-left: w510 -> [w563]
          shift-right: [w561] -> _
          shift-left: w510 -> [w560]
          shift-right: [w559] -> _
          shift-left: w510 -> [w558]
          shift-right: [w557] -> _
          shift-left: w510 -> [w556]
          shift-right: [w555] -> _
          shift-left: w510 -> [w554]
          shift-right: [w553] -> _
          shift-left: 0 -> [w552]
          shift-right: [w551] -> _
          shift-left: 0 -> [w550]
          shift-right: [w549] -> _
          shift-left: 0 -> [w548]
          shift-right: [w546] -> _
          shift-left: 0 -> [w547]
          shift-right: [w545] -> _
          shift-left: 0 -> [w544]
          shift-right: [w539] -> w503
          shift-left: w520 -> [w570]
          shift-right: [w538] -> w502
          shift-left: w519 -> [w574]
          shift-right: [w537] -> w501
          shift-left: w518 -> [w573]
          shift-right: [w536] -> w500
          shift-left: w517 -> [w572]
          shift-right: [w535] -> w499
          shift-left: w516 -> [w571]
          shift-right: [w534] -> w498
          shift-left: w513 -> [w564]
          shift-right: [w533] -> w497
          shift-left: w514 -> [w565]
          shift-right: [w532] -> w496
          shift-left: w515 -> [w566]
          shift-right: [w531] -> w494
          shift-left: w495 -> [w567]
          shift-right: [w530] -> w492
          shift-left: w493 -> [w568]
          i -> [w541]
          n83 = String Subset(string=w597, offset (0)=w541, length (rest)=1 ("length (rest)")) -> (substring=w569:string)
          n84 = String Subset(string="none11read1Pread2Pread3Pread4Pread5Pread1Tread2Tread3Tread4Tread5T", offset (0)=w540, length (rest)=6 ("length (rest)")) -> (substring=w543:string)
          n85 = case shown="\"read1P\"" w543 {
            tunnel: w569 -> [w632 w666 w722 w776 w843 w902 w963 w1022 w1081 w1140 w1199]
            tunnel: [w629 w669 w724 w783 w829 w905 w966 w1025 w1084 w1143 w1202] -> w595
            tunnel: [w628 w664 w726 w788 w841 w895 w958 w1017 w1076 w1135 w1194] -> w594
            tunnel: w593 -> [w628 w665 w726 w788 w841 w895 w958 w1017 w1076 w1135 w1194]
            tunnel: w592 -> [w625 w667 w721 w771 w847 w899 w962 w1021 w1080 w1139 w1198]
            tunnel: [w625 w670 w721 w771 w847 w899 w962 w1021 w1080 w1139 w1198] -> w591
            tunnel: w590 -> [w626 w663 w731 w784 w839 w898 w961 w1020 w1079 w1138 w1197]
            tunnel: [w626 w663 w730 w784 w839 w898 w961 w1020 w1079 w1138 w1197] -> w589
            tunnel: w588 -> [w627 w659 w709 w787 w840 w894 w957 w1016 w1075 w1134 w1193]
            tunnel: [w627 w659 w729 w787 w840 w894 w957 w1016 w1075 w1134 w1193] -> w585
            tunnel: w540 -> [_ w668 w725 w768 w844 w904 w965 w1024 w1083 w1142 w1201]
            tunnel: w587 -> [w622 w658 w723 w789 w836 w893 w956 w1015 w1074 w1133 w1192]
            tunnel: [w622 w658 w723 w780 w836 w893 w956 w1015 w1074 w1133 w1192] -> w586
            tunnel: w584 -> [w619 w662 w720 w786 w838 w897 w960 w1019 w1078 w1137 w1196]
            tunnel: [w619 w662 w720 w785 w838 w897 w960 w1019 w1078 w1137 w1196] -> w583
            tunnel: w582 -> [w620 w661 w719 w779 w849 w896 w959 w1018 w1077 w1136 w1195]
            tunnel: w581 -> [w621 w660 w718 w778 w837 w907 w950 w1009 w1061 w1120 w1179]
            tunnel: w580 -> [w624 w657 w717 w782 w828 w892 w955 w1014 w1073 w1132 w1191]
            tunnel: [w624 w657 w717 w782 w842 w892 w955 w1014 w1073 w1132 w1191] -> w579
            tunnel: w578 -> [w623 w656 w716 w781 w835 w901 w947 w998 w1058 w1114 w1176]
            tunnel: [w623 w656 w716 w781 w835 w900 w947 w998 w1058 w1114 w1176] -> w577
            tunnel: [w621 w660 w718 w778 w837 w906 w950 w1009 w1061 w1120 w1179] -> w576
            tunnel: [w620 w661 w719 w779 w848 w896 w959 w1018 w1077 w1136 w1195] -> w575
            tunnel: [w614 w655 w713 w769 w830 w891 w954 w1013 w1072 w1131 w1190] -> w539
            tunnel: w570 -> [w614 w654 w713 w769 w830 w891 w954 w1013 w1072 w1131 w1190]
            tunnel: [w618 w653 w715 w775 w834 w886 w951 w1010 w1069 w1128 w1187] -> w538
            tunnel: w574 -> [w618 w653 w714 w775 w834 w886 w951 w1010 w1069 w1128 w1187]
            tunnel: [w617 w652 w710 w774 w831 w889 w953 w1012 w1071 w1130 w1189] -> w537
            tunnel: w573 -> [w617 w652 w710 w773 w831 w889 w953 w1012 w1071 w1130 w1189]
            tunnel: [w616 w651 w712 w772 w833 w887 w952 w1011 w1070 w1129 w1188] -> w536
            tunnel: w572 -> [w616 w651 w712 w772 w832 w887 w952 w1011 w1070 w1129 w1188]
            tunnel: [w615 w650 w711 w770 w812 w890 w943 w993 w1067 w1127 w1186] -> w535
            tunnel: w571 -> [w615 w650 w711 w770 w812 w888 w943 w993 w1067 w1127 w1186]
            tunnel: w568 -> [w609 w645 w704 w763 w823 w881 w931 w989 w1062 w1121 w1185]
            tunnel: w567 -> [w610 w646 w705 w764 w824 w882 w932 w990 w1064 w1126 w1180]
            tunnel: w566 -> [w611 w647 w706 w765 w825 w883 w933 w991 w1068 w1123 w1181]
            tunnel: w565 -> [w612 w648 w707 w766 w826 w884 w934 w995 w1065 w1124 w1182]
            tunnel: w564 -> [w613 w649 w708 w767 w827 w885 w944 w994 w1066 w1125 w1183]
            tunnel: [w613 w649 w708 w767 w827 w885 w942 w994 w1066 w1125 w1183] -> w534
            tunnel: [w612 w648 w707 w766 w826 w884 w934 w992 w1065 w1124 w1182] -> w533
            tunnel: [w611 w647 w706 w765 w825 w883 w933 w991 w1063 w1123 w1181] -> w532
            tunnel: [w610 w646 w705 w764 w824 w882 w932 w990 w1064 w1122 w1180] -> w531
            tunnel: [w609 w645 w704 w763 w823 w881 w931 w989 w1062 w1121 w1184] -> w530
            tunnel: w563 -> [w608 w644 w703 w762 w822 w880 w949 w1006 w1055 w1117 w1166]
            tunnel: [w608 w644 w703 w762 w822 w880 w948 w1006 w1055 w1117 w1166] -> w562
            tunnel: [w607 w643 w702 w761 w821 w879 w941 w1007 w1054 w1116 w1167] -> w561
            tunnel: w560 -> [w607 w643 w702 w761 w821 w879 w941 w1008 w1054 w1116 w1167]
            tunnel: [w606 w642 w701 w760 w820 w878 w940 w1005 w1059 w1115 w1168] -> w559
            tunnel: w558 -> [w606 w642 w701 w760 w820 w878 w940 w1005 w1060 w1115 w1168]
            tunnel: [w605 w641 w700 w759 w819 w877 w939 w1004 w1053 w1119 w1169] -> w557
            tunnel: w556 -> [w605 w641 w700 w759 w819 w877 w939 w1004 w1053 w1118 w1169]
            tunnel: [w604 w640 w699 w758 w818 w876 w938 w1003 w1052 w1110 w1178] -> w555
            tunnel: w554 -> [w604 w640 w699 w758 w818 w876 w938 w1003 w1052 w1110 w1177]
            tunnel: [w603 w639 w698 w757 w817 w875 w945 w1002 w1051 w1111 w1170] -> w553
            tunnel: w552 -> [w603 w639 w698 w757 w817 w875 w946 w1002 w1051 w1111 w1170]
            tunnel: [w602 w638 w697 w756 w816 w874 w937 w997 w1050 w1109 w1171] -> w551
            tunnel: w550 -> [w602 w638 w697 w756 w816 w874 w937 w996 w1050 w1109 w1171]
            tunnel: [w601 w637 w696 w755 w815 w873 w936 w1001 w1057 w1108 w1172] -> w549
            tunnel: w548 -> [w601 w637 w696 w755 w815 w873 w936 w1001 w1056 w1108 w1172]
            tunnel: w547 -> [w600 w636 w695 w754 w814 w872 w935 w1000 w1049 w1112 w1173]
            tunnel: [w600 w636 w695 w754 w814 w872 w935 w1000 w1049 w1113 w1173] -> w546
            tunnel: [w599 w635 w694 w753 w813 w871 w930 w999 w1048 w1107 w1175] -> w545
            tunnel: w544 -> [w599 w635 w694 w753 w813 w871 w930 w999 w1048 w1107 w1174]
            frame "none11", Default {
              n86 = Equal?(x=w632, y="a") -> (x = y?=w630:bool)
              n87 = case shown="False" w630 {
                tunnel: [0 6] -> w629
                frame False {
                }
                frame True {
                  # "Go to read1P"
                }
              }
            }
            frame "read1P" {
              n88 = Equal?(x=w666, y="b") -> (x = y?=w671:bool)
              n89 = case shown="True" w671 {
                tunnel: [w681 0] -> w664
                tunnel: w667 -> [w675 w689]
                tunnel: [w679 w689] -> w670
                tunnel: w666 -> [w678 _]
                tunnel: [w676 12] -> w669
                tunnel: w668 -> [w676 _]
                tunnel: w665 -> [w674 w688]
                tunnel: [w673 w686] -> w655
                tunnel: w654 -> [w673 _]
                frame False {
                  n90 = String To Byte Array(string=w678) -> (unsigned byte array=w677:u8[])
                  n91 = Insert Into Array(array=w675, index=w674, new element=w677) -> (w679:dbl[])
                  n92 = Add(x=w674, y=1) -> (x+y=w681:i32)
                }
                frame True {
                  # "Go to read2P"
                  n93 = Byte Array To String(unsigned byte array=w689) -> (string=w690:string)
                  n94 = String Subset(string=w690, offset (0)=0, length (rest)=w688) -> (substring=w687:string)
                  n95 = Fract/Exp String To Number(string=w687) -> (number=w685:dbl)  [unwired: 3 in, 1 out]
                  n96 = Multiply(x=w685, y="Servo 1 Position Slope") -> (x*y=w684:dbl)
                  n97 = Add(x=w684, y="Servo 1 Position Intercept") -> (x+y=w686:dbl)
                  "Pos1 number" <- w686
                }
              }
            }
            frame "read2P" {
              n98 = Equal?(x=w722, y="c") -> (x = y?=w727:bool)
              n99 = case shown="True" w727 {
                tunnel: [w740 0] -> w729
                tunnel: w709 -> [w734 w749]
                tunnel: w731 -> [w738 w747]
                tunnel: [w737 w747] -> w730
                tunnel: w722 -> [w736 _]
                tunnel: [w733 18] -> w724
                tunnel: w725 -> [w733 _]
                tunnel: [w732 w743] -> w715
                tunnel: w714 -> [w732 _]
                frame False {
                  n100 = String To Byte Array(string=w736) -> (unsigned byte array=w735:u8[])
                  n101 = Insert Into Array(array=w738, index=w734, new element=w735) -> (w737:dbl[])
                  n102 = Add(x=w734, y=1) -> (x+y=w740:i32)
                }
                frame True {
                  # "Go to read3P"
                  n103 = Byte Array To String(unsigned byte array=w747) -> (string=w746:string)
                  n104 = String Subset(string=w746, offset (0)=0, length (rest)=w749) -> (substring=w748:string)
                  n105 = Fract/Exp String To Number(string=w748) -> (number=w744:dbl)  [unwired: 3 in, 1 out]
                  n106 = Multiply(x=w744, y="Servo 2 Position Slope") -> (x*y=w745:dbl)
                  n107 = Add(x=w745, y="Servo 2 Position Intercept") -> (x+y=w743:dbl)
                  "Pos2 number" <- w743
                }
              }
            }
            frame "read3P" {
              n108 = Equal?(x=w776, y="d") -> (x = y?=w790:bool)
              n109 = case shown="True" w790 {
                tunnel: [w799 0] -> w780
                tunnel: w789 -> [w793 w806]
                tunnel: w786 -> [w797 w807]
                tunnel: [w796 w807] -> w785
                tunnel: w776 -> [w795 _]
                tunnel: [w792 24] -> w783
                tunnel: w768 -> [w792 _]
                tunnel: [w791 w800] -> w774
                tunnel: w773 -> [w791 _]
                frame False {
                  n110 = String To Byte Array(string=w795) -> (unsigned byte array=w794:u8[])
                  n111 = Insert Into Array(array=w797, index=w793, new element=w794) -> (w796:dbl[])
                  n112 = Add(x=w793, y=1) -> (x+y=w799:i32)
                }
                frame True {
                  # "Go to read4P"
                  n113 = Byte Array To String(unsigned byte array=w807) -> (string=w808:string)
                  n114 = String Subset(string=w808, offset (0)=0, length (rest)=w806) -> (substring=w805:string)
                  n115 = Fract/Exp String To Number(string=w805) -> (number=w803:dbl)  [unwired: 3 in, 1 out]
                  n116 = Multiply(x=w803, y="Servo 3 Position Slope") -> (x*y=w804:dbl)
                  n117 = Add(x=w804, y="Servo 3 Position Intercept") -> (x+y=w800:dbl)
                  "Pos3 number" <- w800
                }
              }
            }
            frame "read4P" {
              n118 = Equal?(x=w843, y="e") -> (x = y?=w845:bool)
              n119 = case shown="True" w845 {
                tunnel: [w858 0] -> w842
                tunnel: w828 -> [w852 w866]
                tunnel: w849 -> [w856 w867]
                tunnel: [w855 w867] -> w848
                tunnel: w843 -> [w854 _]
                tunnel: [w851 30] -> w829
                tunnel: w844 -> [w851 _]
                tunnel: [w850 w863] -> w833
                tunnel: w832 -> [w850 _]
                frame False {
                  n120 = String To Byte Array(string=w854) -> (unsigned byte array=w853:u8[])
                  n121 = Insert Into Array(array=w856, index=w852, new element=w853) -> (w855:dbl[])
                  n122 = Add(x=w852, y=1) -> (x+y=w858:i32)
                }
                frame True {
                  # "Go to read5P"
                  n123 = Byte Array To String(unsigned byte array=w867) -> (string=w868:string)
                  n124 = String Subset(string=w868, offset (0)=0, length (rest)=w866) -> (substring=w865:string)
                  n125 = Fract/Exp String To Number(string=w865) -> (number=w862:dbl)  [unwired: 3 in, 1 out]
                  n126 = Multiply(x=w862, y="Servo 4 Position Slope") -> (x*y=w864:dbl)
                  n127 = Add(x=w864, y="Servo 4 Position Intercept") -> (x+y=w863:dbl)
                  "Pos4 number" <- w863
                }
              }
            }
            frame "read5P" {
              n128 = Equal?(x=w902, y="v") -> (x = y?=w903:bool)
              n129 = case shown="True" w903 {
                tunnel: [w917 0] -> w900
                tunnel: w901 -> [w911 w924]
                tunnel: w907 -> [w915 w925]
                tunnel: [w914 w925] -> w906
                tunnel: w902 -> [w913 _]
                tunnel: [w910 36] -> w905
                tunnel: w904 -> [w910 _]
                tunnel: [w909 w919] -> w890
                tunnel: w888 -> [w909 _]
                frame False {
                  n130 = String To Byte Array(string=w913) -> (unsigned byte array=w912:u8[])
                  n131 = Insert Into Array(array=w915, index=w911, new element=w912) -> (w914:dbl[])
                  n132 = Add(x=w911, y=1) -> (x+y=w917:i32)
                }
                frame True {
                  # "Go to read1T"
                  n133 = Byte Array To String(unsigned byte array=w925) -> (string=w926:string)
                  n134 = String Subset(string=w926, offset (0)=0, length (rest)=w924) -> (substring=w923:string)
                  n135 = Fract/Exp String To Number(string=w923) -> (number=w921:dbl)  [unwired: 3 in, 1 out]
                  n136 = Multiply(x=w921, y="Servo 5 Position Slope") -> (x*y=w922:dbl)
                  n137 = Add(x=w922, y="Servo 5 Position Intercept") -> (x+y=w919:dbl)
                  "Pos5 number" <- w919
                }
              }
            }
            frame "read1T" {
              n138 = Equal?(x=w963, y="w") -> (x = y?=w964:bool)
              n139 = case shown="True" w964 {
                tunnel: [w976 0] -> w945
                tunnel: w946 -> [w970 w982]
                tunnel: w949 -> [w974 w984]
                tunnel: [w973 w984] -> w948
                tunnel: w963 -> [w972 _]
                tunnel: [w969 42] -> w966
                tunnel: w965 -> [w969 _]
                tunnel: [w968 w979] -> w942
                tunnel: w944 -> [w968 _]
                frame False {
                  n140 = String To Byte Array(string=w972) -> (unsigned byte array=w971:u8[])
                  n141 = Insert Into Array(array=w974, index=w970, new element=w971) -> (w973:dbl[])
                  n142 = Add(x=w970, y=1) -> (x+y=w976:i32)
                }
                frame True {
                  # "Go to read2T"
                  n143 = Byte Array To String(unsigned byte array=w984) -> (string=w985:string)
                  n144 = String Subset(string=w985, offset (0)=0, length (rest)=w982) -> (substring=w983:string)
                  n145 = Fract/Exp String To Number(string=w983) -> (number=w980:dbl)  [unwired: 3 in, 1 out]
                  n146 = Multiply(x=w980, y="Servo 1 Torque Slope") -> (x*y=w981:dbl)
                  n147 = Add(x=w981, y="Servo 1 Torque Intercept") -> (x+y=w979:dbl)
                  "Torq1 number" <- w979
                }
              }
            }
            frame "read2T" {
              n148 = Equal?(x=w1022, y="x") -> (x = y?=w1023:bool)
              n149 = case shown="True" w1023 {
                tunnel: [w1035 0] -> w997
                tunnel: w996 -> [w1029 w1041]
                tunnel: w1008 -> [w1033 w1043]
                tunnel: [w1032 w1043] -> w1007
                tunnel: w1022 -> [w1031 _]
                tunnel: [w1028 48] -> w1025
                tunnel: w1024 -> [w1028 _]
                tunnel: [w1027 w1038] -> w992
                tunnel: w995 -> [w1027 _]
                frame False {
                  n150 = String To Byte Array(string=w1031) -> (unsigned byte array=w1030:u8[])
                  n151 = Insert Into Array(array=w1033, index=w1029, new element=w1030) -> (w1032:dbl[])
                  n152 = Add(x=w1029, y=1) -> (x+y=w1035:i32)
                }
                frame True {
                  # "Go to read3T"
                  n153 = Byte Array To String(unsigned byte array=w1043) -> (string=w1044:string)
                  n154 = String Subset(string=w1044, offset (0)=0, length (rest)=w1041) -> (substring=w1042:string)
                  n155 = Fract/Exp String To Number(string=w1042) -> (number=w1039:dbl)  [unwired: 3 in, 1 out]
                  n156 = Multiply(x=w1039, y="Servo 2 Torque Slope") -> (x*y=w1040:dbl)
                  n157 = Add(x=w1040, y="Servo 2 Torque Intercept") -> (x+y=w1038:dbl)
                  "Torq2 number" <- w1038
                }
              }
            }
            frame "read3T" {
              n158 = Equal?(x=w1081, y="y") -> (x = y?=w1082:bool)
              n159 = case shown="True" w1082 {
                tunnel: [w1094 0] -> w1057
                tunnel: w1056 -> [w1088 w1100]
                tunnel: w1060 -> [w1092 w1102]
                tunnel: [w1091 w1102] -> w1059
                tunnel: w1081 -> [w1090 _]
                tunnel: [w1087 54] -> w1084
                tunnel: w1083 -> [w1087 _]
                tunnel: [w1086 w1098] -> w1063
                tunnel: w1068 -> [w1086 _]
                frame False {
                  n160 = String To Byte Array(string=w1090) -> (unsigned byte array=w1089:u8[])
                  n161 = Insert Into Array(array=w1092, index=w1088, new element=w1089) -> (w1091:dbl[])
                  n162 = Add(x=w1088, y=1) -> (x+y=w1094:i32)
                }
                frame True {
                  # "Go to read4T"
                  n163 = Byte Array To String(unsigned byte array=w1102) -> (string=w1103:string)
                  n164 = String Subset(string=w1103, offset (0)=0, length (rest)=w1100) -> (substring=w1101:string)
                  n165 = Fract/Exp String To Number(string=w1101) -> (number=w1097:dbl)  [unwired: 3 in, 1 out]
                  n166 = Multiply(x=w1097, y="Servo 3 Torque Slope") -> (x*y=w1099:dbl)
                  n167 = Add(x=w1099, y="Servo 3 Torque Intercept") -> (x+y=w1098:dbl)
                  "Torq3 number" <- w1098
                }
              }
            }
            frame "read4T" {
              n168 = Equal?(x=w1140, y="z") -> (x = y?=w1141:bool)
              n169 = case shown="True" w1141 {
                tunnel: [w1153 0] -> w1113
                tunnel: w1112 -> [w1147 w1159]
                tunnel: w1118 -> [w1151 w1161]
                tunnel: [w1150 w1161] -> w1119
                tunnel: w1140 -> [w1149 _]
                tunnel: [w1146 60] -> w1143
                tunnel: w1142 -> [w1146 _]
                tunnel: [w1145 w1156] -> w1122
                tunnel: w1126 -> [w1145 _]
                frame False {
                  n170 = String To Byte Array(string=w1149) -> (unsigned byte array=w1148:u8[])
                  n171 = Insert Into Array(array=w1151, index=w1147, new element=w1148) -> (w1150:dbl[])
                  n172 = Add(x=w1147, y=1) -> (x+y=w1153:i32)
                }
                frame True {
                  # "Go to read5T"
                  n173 = Byte Array To String(unsigned byte array=w1161) -> (string=w1162:string)
                  n174 = String Subset(string=w1162, offset (0)=0, length (rest)=w1159) -> (substring=w1160:string)
                  n175 = Fract/Exp String To Number(string=w1160) -> (number=w1157:dbl)  [unwired: 3 in, 1 out]
                  n176 = Multiply(x=w1157, y="Servo 4 Torque Slope") -> (x*y=w1158:dbl)
                  n177 = Add(x=w1158, y="Servo 4 Torque Intercept") -> (x+y=w1156:dbl)
                  "Torq4 number" <- w1156
                }
              }
            }
            frame "read5T" {
              n178 = Equal?(x=w1199, y="!") -> (x = y?=w1200:bool)
              n179 = case shown="True" w1200 {
                tunnel: [w1212 0] -> w1175
                tunnel: w1174 -> [w1206 w1218]
                tunnel: w1177 -> [w1210 w1220]
                tunnel: [w1209 w1220] -> w1178
                tunnel: w1199 -> [w1208 _]
                tunnel: [w1205 0] -> w1202
                tunnel: w1201 -> [w1205 _]
                tunnel: [w1204 w1213] -> w1184
                tunnel: w1185 -> [w1204 _]
                frame False {
                  n180 = String To Byte Array(string=w1208) -> (unsigned byte array=w1207:u8[])
                  n181 = Insert Into Array(array=w1210, index=w1206, new element=w1207) -> (w1209:dbl[])
                  n182 = Add(x=w1206, y=1) -> (x+y=w1212:i32)
                }
                frame True {
                  # "Go to none11"
                  n183 = Byte Array To String(unsigned byte array=w1220) -> (string=w1221:string)
                  n184 = String Subset(string=w1221, offset (0)=0, length (rest)=w1218) -> (substring=w1219:string)
                  n185 = Fract/Exp String To Number(string=w1219) -> (number=w1216:dbl)  [unwired: 3 in, 1 out]
                  n186 = Multiply(x=w1216, y="Servo 5 Torque Slope") -> (x*y=w1217:dbl)
                  n187 = Add(x=w1217, y="Servo 5 Torque Intercept") -> (x+y=w1213:dbl)
                  "Torq5 number" <- w1213
                }
              }
            }
          }
        }
      }
    }
    n188 = call-poly <vilib>:"Mean.vi"("X"=w110) -> ("mean"=w71:dbl)  [unwired: 1 out]
    "Calculated Time Delay" <- w71
    n189 = Bundle(0, "mean"=w71, w387) -> (→"Bytes at port":cluster{i32, "mean":dbl, dbl[]})  [unwired: 1 in]
    n190 = Subtract(x=w84, y=1) -> (x-y=w330:i32)
    n191 = Subtract(x=w84, y=1) -> (x-y=w319:i32)
    n192 = Subtract(x=w84, y=1) -> (x-y=w322:i32)
    n193 = Subtract(x=w84, y=1) -> (x-y=w313:i32)
    n194 = Subtract(x=w84, y=1) -> (x-y=w316:i32)
    n195 = Index Array(array=w317, index=w319) -> (element=w301:dbl)
    n196 = Index Array(array=w320, index=w322) -> (element=w306:dbl)
    n197 = Index Array(array=w314, index=w316) -> (element=w295:dbl)
    n198 = Index Array(array=w284, index=w313) -> (element=w286:dbl)
    n199 = Index Array(array=w328, index=w330) -> (element=w325:dbl)
    n200 = Less?(x=w289, y="Lowest Servo Angle") -> (x < y?=w290:bool)
    n201 = Greater?(x=w289, y="Highest Servo Angle") -> (0:w292:bool)
    n202 = Or(x=w292, y=w290) -> (x .or. y?=w291:bool)
    n203 = case shown="True" w291 {
      tunnel: w286 -> [_ w464]
      tunnel: w289 -> [w462 _]
      tunnel: [w462 w464] -> w285
      tunnel: [FALSE TRUE] -> w234
      frame False {
      }
      frame True {
      }
    }
    n204 = Greater?(x=w293, y="Highest Servo Angle") -> (0:w296:bool)
    n205 = Less?(x=w293, y="Lowest Servo Angle") -> (x < y?=w297:bool)
    n206 = Or(x=w296, y=w297) -> (x .or. y?=w298:bool)
    n207 = case shown="True" w298 {
      tunnel: w295 -> [_ w468]
      tunnel: w293 -> [w466 _]
      tunnel: [w466 w468] -> w294
      tunnel: [FALSE TRUE] -> w235
      frame False {
      }
      frame True {
      }
    }
    n208 = Or(x=w235, y=w234) -> (x .or. y?=w232:bool)
    n209 = Greater?(x=w299, y="Highest Servo Angle") -> (0:w304:bool)
    n210 = Less?(x=w299, y="Lowest Servo Angle") -> (x < y?=w302:bool)
    n211 = Or(x=w304, y=w302) -> (x .or. y?=w303:bool)
    n212 = Tick Count (ms)() -> (millisecond timer value=w153:u32)
    n213 = case shown="True" w303 {
      tunnel: w301 -> [_ w472]
      tunnel: w299 -> [w470 _]
      tunnel: [w470 w472] -> w300
      tunnel: [FALSE TRUE] -> w233
      frame False {
      }
      frame True {
      }
    }
    n214 = Divide(x=w153, y=1000) -> (x/y=w151:dbl)
    n215 = Or(x=w233, y=w232) -> (x .or. y?=w230:bool)
    n216 = Sine(x=w151) -> (sin(x)=w142:dbl)
    n217 = Greater?(x=w305, y="Highest Servo Angle") -> (0:w310:bool)
    n218 = Less?(x=w305, y="Lowest Servo Angle") -> (x < y?=w308:bool)
    n219 = Or(x=w310, y=w308) -> (x .or. y?=w309:bool)
    n220 = case shown="True" w309 {
      tunnel: w306 -> [_ w476]
      tunnel: w305 -> [w474 _]
      tunnel: [w474 w476] -> w307
      tunnel: [FALSE TRUE] -> w231
      frame False {
      }
      frame True {
      }
    }
    n221 = Multiply(x=2, y=w142) -> (x*y=w144:dbl)
    n222 = Or(x=w231, y=w230) -> (x .or. y?=w228:bool)
    n223 = Multiply(x=w142, y=0.1) -> (x*y=w143:dbl)
    n224 = Less?(x=w323, y="Lowest Servo Angle") -> (x < y?=w324:bool)
    n225 = Greater?(x=w323, y="Highest Servo Angle") -> (0:w327:bool)
    n226 = Or(x=w327, y=w324) -> (x .or. y?=w326:bool)
    n227 = Insert Into Array(array=w146, index=w84, new element=w144) -> (w73:dbl[])
    n228 = Insert Into Array(array=w145, index=w84, new element=w143) -> (w72:dbl[])
    n229 = Insert Into Array(array=w147, index=w84, new element=w142) -> (w89:dbl[])
    n230 = case shown="True" w326 {
      tunnel: w325 -> [_ w480]
      tunnel: w323 -> [w478 _]
      tunnel: [w478 w480] -> w311
      tunnel: [FALSE TRUE] -> w229
      frame False {
      }
      frame True {
      }
    }
    n231 = call <vilib>:"Amplitude and Phase Spectrum.vi"("dt"=w71, "Signal (V)"=w89) -> ("df"=w69:dbl, "Amp Spectrum Mag (Vrms)"=w62:dbl[])  [unwired: 1 in, 1 out]
    n232 = call <vilib>:"Amplitude and Phase Spectrum.vi"("dt"=w71, "Signal (V)"=w73) -> ("df"=w68:dbl, "Amp Spectrum Mag (Vrms)"=w67:dbl[])  [unwired: 1 in, 1 out]
    n233 = Or(x=w229, y=w228) -> (x .or. y?=→"Minimum or Maximum Angle Exceeded":bool)
    n234 = call <vilib>:"Amplitude and Phase Spectrum.vi"("dt"=w71, "Signal (V)"=w72) -> ("df"=w64:dbl, "Amp Spectrum Mag (Vrms)"=w63:dbl[])  [unwired: 1 in, 1 out]
    n235 = Insert Into Array(array=w328, index=w84, new element=w311) -> (w92:dbl[])
    n236 = Insert Into Array(array=w320, index=w84, new element=w307) -> (w94:dbl[])
    n237 = Insert Into Array(array=w284, index=w84, new element=w285) -> (w108:dbl[])
    n238 = Insert Into Array(array=w317, index=w84, new element=w300) -> (w98:dbl[])
    n239 = Insert Into Array(array=w314, index=w84, new element=w294) -> (w102:dbl[])
    n240 = Bundle("timeout (s)"=w65, "df"=w69, "Amp Spectrum Mag (Vrms)"=w62) -> (→"Lift FFT":T3)  [unwired: 1 in]
    n241 = Bundle("timeout (s)"=w65, "df"=w64, "Amp Spectrum Mag (Vrms)"=w63) -> (→"Yaw FFT":T3)  [unwired: 1 in]
    n242 = Bundle("timeout (s)"=w65, "df"=w68, "Amp Spectrum Mag (Vrms)"=w67) -> (→"Drag FFT":T3)  [unwired: 1 in]
    n243 = Greater?(x=w214, y="Max Torque") -> (0:w208:bool)
    n244 = Greater?(x=w210, y="Max Torque") -> (0:w207:bool)
    n245 = Greater?(x=w211, y="Max Torque") -> (0:w206:bool)
    n246 = Or(x=w207, y=w208) -> (x .or. y?=w205:bool)
    n247 = Greater?(x=w212, y="Max Torque") -> (0:w204:bool)
    n248 = Subtract(x=w182, y=w186) -> (x-y=w187:dbl)
    n249 = Subtract(x=w183, y=w186) -> (x-y=w188:dbl)
    n250 = Or(x=w206, y=w205) -> (x .or. y?=w201:bool)
    n251 = Greater?(x=w213, y="Max Torque") -> (0:w203:bool)
    n252 = Subtract(x=w181, y=w186) -> (x-y=w189:dbl)
    n253 = Subtract(x=w184, y=w186) -> (x-y=w190:dbl)
    n254 = Or(x=w204, y=w201) -> (x .or. y?=w202:bool)
    n255 = Bundle(w136, 20, 0.5, 0.1, w136) -> (w140:cluster{i32, i32, dbl, dbl, i32})  [unwired: 1 in]
    n256 = Subtract(x=w185, y=w186) -> (x-y=w191:dbl)
    n257 = Bundle(w132, 1, 0.1, 0.05, w132) -> (w131:cluster{i32, i32, dbl, dbl, i32})  [unwired: 1 in]
    n258 = Insert Into Array(array=w339, index=w84, new element=w214) -> (w226:dbl[])
    n259 = Insert Into Array(array=w338, index=w84, new element=w210) -> (w224:dbl[])
    n260 = Insert Into Array(array=w335, index=w84, new element=w213) -> (w225:dbl[])
    n261 = Or(x=w203, y=w202) -> (x .or. y?=→"Maximum Torque Exceeded":bool)
    n262 = Insert Into Array(array=w337, index=w84, new element=w211) -> (w223:dbl[])
    n263 = Insert Into Array(array=w336, index=w84, new element=w212) -> (w222:dbl[])
    n264 = Build Array(w191, w190, w189, w188, w187) -> (w156:dbl[])
    "Output Angles" <- w156
    n265 = property on="Lift FFT" class="WFGraph (strict)"("XScale.Range"=w140) -> ()  [unwired: 2 in, 2 out]
    n266 = property on="Lift FFT" class="WFGraph (strict)"("YScale.Range"=w131) -> ()  [unwired: 2 in, 2 out]
    n267 = call "PlotSubArray.vi"("Time Step (s)"=w71, "Plot Last x Seconds"="Plot Last x Seconds", "Iteration"=w84, "Array"=w102) -> ("Sub Array"=w77:dbl[], "Time Offset"=w100:dbl)  [unwired: 6 in]
    n268 = call "PlotSubArray.vi"("Time Step (s)"=w71, "Plot Last x Seconds"="Plot Last x Seconds", "Iteration"=w84, "Array"=w93) -> ("Sub Array"=w83:dbl[])  [unwired: 6 in, 1 out]
    n269 = call "PlotSubArray.vi"("Time Step (s)"=w71, "Plot Last x Seconds"="Plot Last x Seconds", "Iteration"=w84, "Array"=w101) -> ("Sub Array"=w76:dbl[])  [unwired: 6 in, 1 out]
    n270 = call "PlotSubArray.vi"("Time Step (s)"=w71, "Plot Last x Seconds"="Plot Last x Seconds", "Iteration"=w84, "Array"=w94) -> ("Sub Array"=w81:dbl[], "Time Offset"=w96:dbl)  [unwired: 6 in]
    n271 = call "PlotSubArray.vi"("Time Step (s)"=w71, "Plot Last x Seconds"="Plot Last x Seconds", "Iteration"=w84, "Array"=w95) -> ("Sub Array"=w80:dbl[])  [unwired: 6 in, 1 out]
    n272 = call "PlotSubArray.vi"("Time Step (s)"=w71, "Plot Last x Seconds"="Plot Last x Seconds", "Iteration"=w84, "Array"=w99) -> ("Sub Array"=w79:dbl[])  [unwired: 6 in, 1 out]
    n273 = call "PlotSubArray.vi"("Time Step (s)"=w71, "Plot Last x Seconds"="Plot Last x Seconds", "Iteration"=w84, "Array"=w98) -> ("Sub Array"=w78:dbl[], "Time Offset"=w97:dbl)  [unwired: 6 in]
    n274 = call "PlotSubArray.vi"("Time Step (s)"=w71, "Plot Last x Seconds"="Plot Last x Seconds", "Iteration"=w84, "Array"=w109) -> ("Sub Array"=w74:dbl[])  [unwired: 6 in, 1 out]
    n275 = call "PlotSubArray.vi"("Time Step (s)"=w71, "Plot Last x Seconds"="Plot Last x Seconds", "Iteration"=w84, "Array"=w108) -> ("Sub Array"=w75:dbl[], "Time Offset"=w107:dbl)  [unwired: 6 in]
    n276 = call "PlotSubArray.vi"("Time Step (s)"=w71, "Plot Last x Seconds"="Plot Last x Seconds", "Iteration"=w84, "Array"=w92) -> ("Sub Array"=w82:dbl[], "Time Offset"=w91:dbl)  [unwired: 6 in]
    n277 = Divide(x="Length of Segments", y=100) -> (x/y=w167:dbl)
    n278 = Initialize Array(0.0 ("element"), 1 ("dimension size")) -> (w194:dbl[])
    n279 = Initialize Array(0.0 ("element"), 1 ("dimension size")) -> (w193:dbl[])
    n280 = Build Array(w79, w78) -> (w354:dbl[][])
    n281 = Build Array(w74, w75) -> (w106:dbl[][])
    n282 = Build Array(w76, w77) -> (w104:dbl[][])
    n283 = Build Array(w83, w82) -> (w356:dbl[][])
    n284 = call "PlotSubArray.vi"("Time Step (s)"=w71, "Plot Last x Seconds"="Plot Last x Seconds", "Iteration"=w84, "Array"=w226) -> ("Sub Array"=w221:dbl[], "Time Offset"=w61:dbl)  [unwired: 6 in]
    n285 = Build Array(w80, w81) -> (w355:dbl[][])
    n286 = call "PlotSubArray.vi"("Time Step (s)"=w71, "Plot Last x Seconds"="Plot Last x Seconds", "Iteration"=w84, "Array"=w224) -> ("Sub Array"=w220:dbl[])  [unwired: 6 in, 1 out]
    n287 = call "PlotSubArray.vi"("Time Step (s)"=w71, "Plot Last x Seconds"="Plot Last x Seconds", "Iteration"=w84, "Array"=w223) -> ("Sub Array"=w219:dbl[])  [unwired: 6 in, 1 out]
    n288 = call "PlotSubArray.vi"("Time Step (s)"=w71, "Plot Last x Seconds"="Plot Last x Seconds", "Iteration"=w84, "Array"=w222) -> ("Sub Array"=w218:dbl[])  [unwired: 6 in, 1 out]
    n289 = call "PlotSubArray.vi"("Time Step (s)"=w71, "Plot Last x Seconds"="Plot Last x Seconds", "Iteration"=w84, "Array"=w225) -> ("Sub Array"=w217:dbl[])  [unwired: 6 in, 1 out]
    n290 = Bundle("Time Offset"=w100, "mean"=w71, w104) -> (→"Servo 4 Position":cluster{" Time Offset":dbl, "mean":dbl, dbl[][]})  [unwired: 1 in]
    n291 = Bundle("Time Offset"=w97, "mean"=w71, w354) -> (→"Servo 3 Position":cluster{" Time Offset":dbl, "mean":dbl, dbl[][]})  [unwired: 1 in]
    n292 = Bundle("Time Offset"=w96, "mean"=w71, w355) -> (→"Servo 2 Position":cluster{" Time Offset":dbl, "mean":dbl, dbl[][]})  [unwired: 1 in]
    n293 = Bundle("Time Offset"=w107, "mean"=w71, w106) -> (→"Servo 5 Position":cluster{" Time Offset":dbl, "mean":dbl, dbl[][]})  [unwired: 1 in]
    n294 = Bundle("Time Offset"=w91, "mean"=w71, w356) -> (→"Servo 1 Position":cluster{" Time Offset":dbl, "mean":dbl, dbl[][]})  [unwired: 1 in]
    n295 = Build Array(w221, w220, w219, w218, w217) -> (w216:dbl[][])
    n296 = for {
      N: w115 -> [_]
      shift-right: [w400] -> _
      shift-left: 0.0 -> [w417]
      tunnel: w156 -> [w416]
      shift-right: [w410] -> w163
      shift-left: w194 -> [w398]
      shift-right: [w409] -> w162
      shift-left: w193 -> [w397]
      tunnel: w167 -> [w396]
      i -> [w408]
      (unwired) 100
      # "phi"
      # "L"
      n297 = Index Array(array=w416, index=w408) -> (element=w415:dbl)
      n298 = Index Array(array=w398, index=w408) -> (element=w414:dbl)
      n299 = Index Array(array=w397, index=w408) -> (element=w411:dbl)
      n300 = Divide(x=3.141592653589793, y=180) -> (x/y=w399:dbl)
      n301 = Add(x=w415, y=w417) -> (x+y=w400:dbl)
      n302 = Multiply(x=w399, y=w400) -> (x*y=w402:dbl)
      n303 = Multiply(x=w399, y=w400) -> (x*y=w401:dbl)
      n304 = Increment(x=w408) -> (x+1=w407:i32)
      n305 = Cosine(x=w402) -> (cos(x)=w406:dbl)
      n306 = Sine(x=w401) -> (sin(x)=w405:dbl)
      n307 = Multiply(x=w406, y=w396) -> (x*y=w413:dbl)
      n308 = Multiply(x=w396, y=w405) -> (x*y=w412:dbl)
      n309 = Add(x=w414, y=w413) -> (x+y=w395:dbl)
      n310 = Add(x=w412, y=w411) -> (x+y=w394:dbl)
      n311 = Insert Into Array(array=w398, index=w407, new element=w395) -> (w410:dbl[])
      n312 = Insert Into Array(array=w397, index=w407, new element=w394) -> (w409:dbl[])
    }
    n313 = Bundle("Time Offset"=w61, "mean"=w71, w216) -> (→"Servo Torque":cluster{" Time Offset":dbl, "mean":dbl, dbl[][]})  [unwired: 1 in]
    n314 = call "PlotSubArray.vi"("Time Step (s)"=w71, "Plot Last x Seconds"="Plot Last x Seconds", "Iteration"=w84, "Array"=w89) -> ("Sub Array"=w88:dbl[], "Time Offset"=w85:dbl)  [unwired: 6 in]
    n315 = call "PlotSubArray.vi"("Time Step (s)"=w71, "Plot Last x Seconds"="Plot Last x Seconds", "Iteration"=w84, "Array"=w73) -> ("Sub Array"=w87:dbl[])  [unwired: 6 in, 1 out]
    n316 = call "PlotSubArray.vi"("Time Step (s)"=w71, "Plot Last x Seconds"="Plot Last x Seconds", "Iteration"=w84, "Array"=w72) -> ("Sub Array"=w86:dbl[])  [unwired: 6 in, 1 out]
    n317 = Increment(x=w115) -> (x+1=w180:dbl)
    n318 = Increment(x=w115) -> (x+1=w177:dbl)
    n319 = Increment(x=w115) -> (x+1=w164:dbl)
    n320 = Multiply(x=w180, y="Length of Segments") -> (x*y=w178:dbl)
    n321 = Multiply(x=w177, y="Length of Segments") -> (x*y=w174:dbl)
    n322 = Divide(x="Length of Segments", y=5) -> (x/y=w175:dbl)
    n323 = Divide(x="Length of Segments", y=5) -> (x/y=w176:dbl)
    n324 = Multiply(x=-1, y=w178) -> (x*y=w179:dbl)
    n325 = Build Array(w88, w87, w86) -> (w148:dbl[][])
    n326 = Bundle(w170, w174, w167, w175, w170) -> (w169:cluster{i32, dbl, dbl, dbl, i32})  [unwired: 1 in]
    n327 = for {
      N: w164 -> [_]
      tunnel: w163 -> [w393] mode=indexing
      tunnel: w162 -> [w391] mode=indexing
      tunnel: [w390] -> w160 mode=indexing
      tunnel: [w389] -> w159 mode=indexing
      w392 = 100
      # "Convert nodes from m to cm"
      n328 = Multiply(x=w393, y=w392) -> (x*y=w390:dbl)
      n329 = Multiply(x=w392, y=w391) -> (x*y=w389:dbl)
    }
    n330 = Bundle(w179, w178, w167, w176, w179) -> (w168:cluster{dbl, dbl, dbl, dbl, dbl})  [unwired: 1 in]
    n331 = Bundle("Time Offset"=w85, "mean"=w71, w148) -> (→"Force and Moment Data":cluster{" Time Offset":dbl, "mean":dbl, dbl[][]})  [unwired: 1 in]
    n332 = property on="Waveform" class="XYGraph (strict)"("XScale.Range"=w169) -> ()  [unwired: 2 in, 2 out]
    n333 = property on="Waveform" class="XYGraph (strict)"("YScale.Range"=w168) -> ()  [unwired: 2 in, 2 out]
    n334 = property on="Waveform" class="XYGraph (strict)"("Plot.Point Style"=u8 2) -> ()  [unwired: 2 in, 2 out]
    n335 = Bundle(w160, w159) -> (w158:cluster{dbl[], dbl[]})  [unwired: 1 in]
    n336 = Build Array(w165, w158) -> (→"Waveform":cluster{"X Nodes":dbl[], "Y Nodes":dbl[]}[])
  }
  n337 = VISA Close(VISA resource name=w33, error in (no error)=w32) -> ()  [unwired: 1 out]
  n338 = case shown="True" w34 {
    tunnel: w35 -> [_ w1299]
    tunnel: w31 -> [_ w1298]
    tunnel: w27 -> [_ w1287]
    tunnel: w26 -> [_ w1286]
    tunnel: w25 -> [_ w1285]
    tunnel: w24 -> [_ w1276]
    tunnel: w23 -> [_ w1275]
    tunnel: w22 -> [_ w1274]
    tunnel: w21 -> [_ w1273]
    tunnel: w20 -> [_ w1264]
    tunnel: w19 -> [_ w1263]
    tunnel: w18 -> [_ w1262]
    tunnel: w17 -> [_ w1261]
    tunnel: w16 -> [_ w1259]
    tunnel: w15 -> [_ w1249]
    tunnel: w14 -> [_ w1248]
    tunnel: w13 -> [_ w1247]
    tunnel: w12 -> [_ w1246]
    frame False {
    }
    frame True {
      n339 = call "Convert to Dynamic Data9"("Array"=w1273) -> ("Dynamic Data Type"=w1278:dynamicdata)  [unwired: 3 in]
      n340 = call "Convert to Dynamic Data11"("Array"=w1263) -> ("Dynamic Data Type"=w1270:dynamicdata)  [unwired: 3 in]
      n341 = call "Convert to Dynamic Data13"("Array"=w1261) -> ("Dynamic Data Type"=w1266:dynamicdata)  [unwired: 3 in]
      n342 = call "Convert to Dynamic Data"("Array"=w1298) -> ("Dynamic Data Type"=w1297:dynamicdata)  [unwired: 3 in]
      n343 = call "Convert to Dynamic Data12"("Array"=w1262) -> ("Dynamic Data Type"=w1268:dynamicdata)  [unwired: 3 in]
      n344 = call "Convert to Dynamic Data10"("Array"=w1264) -> ("Dynamic Data Type"=w1272:dynamicdata)  [unwired: 3 in]
      n345 = call "Convert to Dynamic Data17"("Array"=w1247) -> ("Dynamic Data Type"=w1252:dynamicdata)  [unwired: 3 in]
      n346 = call "Convert to Dynamic Data18"("Array"=w1246) -> ("Dynamic Data Type"=w1250:dynamicdata)  [unwired: 3 in]
      n347 = call "Convert to Dynamic Data16"("Array"=w1248) -> ("Dynamic Data Type"=w1254:dynamicdata)  [unwired: 3 in]
      n348 = call "Convert to Dynamic Data15"("Array"=w1249) -> ("Dynamic Data Type"=w1256:dynamicdata)  [unwired: 3 in]
      n349 = call "Convert to Dynamic Data14"("Array"=w1259) -> ("Dynamic Data Type"=w1258:dynamicdata)  [unwired: 3 in]
      n350 = call "Convert to Dynamic Data2"("Array"=w1299) -> ("Dynamic Data Type"=w1296:dynamicdata)  [unwired: 3 in]
      n351 = call "Convert to Dynamic Data6"("Array"=w1276) -> ("Dynamic Data Type"=w1284:dynamicdata)  [unwired: 3 in]
      n352 = call "Convert to Dynamic Data8"("Array"=w1274) -> ("Dynamic Data Type"=w1280:dynamicdata)  [unwired: 3 in]
      n353 = call "Convert to Dynamic Data7"("Array"=w1275) -> ("Dynamic Data Type"=w1282:dynamicdata)  [unwired: 3 in]
      n354 = call "Convert to Dynamic Data5"("Array"=w1287) -> ("Dynamic Data Type"=w1292:dynamicdata)  [unwired: 3 in]
      n355 = call "Convert to Dynamic Data4"("Array"=w1286) -> ("Dynamic Data Type"=w1291:dynamicdata)  [unwired: 3 in]
      n356 = call "Convert to Dynamic Data3"("Array"=w1285) -> ("Dynamic Data Type"=w1293:dynamicdata)  [unwired: 3 in]
      n357 = xnode "Set Dynamic Data Attributes"("Signals In"=w1291, "Signal Name"="Lift Force") -> ("Signals Out"=w1244:dynamicdata)  [unwired: 2 in, 1 out]
      n358 = xnode "Set Dynamic Data Attributes"("Signals In"=w1292, "Signal Name"="Drag Force") -> ("Signals Out"=w1245:dynamicdata)  [unwired: 2 in, 1 out]
      n359 = xnode "Set Dynamic Data Attributes"("Signals In"=w1293, "Signal Name"="Yaw Moment") -> ("Signals Out"=w1243:dynamicdata)  [unwired: 2 in, 1 out]
      n360 = xnode "Set Dynamic Data Attributes"("Signals In"=w1296, "Signal Name"="Servo 1 Commanded Position") -> ("Signals Out"=w1242:dynamicdata)  [unwired: 2 in, 1 out]
      n361 = xnode "Set Dynamic Data Attributes"("Signals In"=w1284, "Signal Name"="Servo 2 Commanded Position") -> ("Signals Out"=w1241:dynamicdata)  [unwired: 2 in, 1 out]
      n362 = xnode "Set Dynamic Data Attributes"("Signals In"=w1280, "Signal Name"="Servo 4 Commanded Position") -> ("Signals Out"=w1239:dynamicdata)  [unwired: 2 in, 1 out]
      n363 = xnode "Set Dynamic Data Attributes"("Signals In"=w1282, "Signal Name"="Servo 3 Commanded Position") -> ("Signals Out"=w1240:dynamicdata)  [unwired: 2 in, 1 out]
      n364 = xnode "Set Dynamic Data Attributes"("Signals In"=w1278, "Signal Name"="Servo 5 Commanded Position") -> ("Signals Out"=w1238:dynamicdata)  [unwired: 2 in, 1 out]
      n365 = xnode "Set Dynamic Data Attributes"("Signals In"=w1297, "Signal Name"="Servo 1 Feedback Position") -> ("Signals Out"=w1237:dynamicdata)  [unwired: 2 in, 1 out]
      n366 = xnode "Set Dynamic Data Attributes"("Signals In"=w1268, "Signal Name"="Servo 1 Feedback Position") -> ("Signals Out"=w1234:dynamicdata)  [unwired: 2 in, 1 out]
      n367 = xnode "Set Dynamic Data Attributes"("Signals In"=w1270, "Signal Name"="Servo 1 Feedback Position") -> ("Signals Out"=w1235:dynamicdata)  [unwired: 2 in, 1 out]
      n368 = xnode "Set Dynamic Data Attributes"("Signals In"=w1252, "Signal Name"="Servo 4  Torque") -> ("Signals Out"=w1229:dynamicdata)  [unwired: 2 in, 1 out]
      n369 = xnode "Set Dynamic Data Attributes"("Signals In"=w1250, "Signal Name"="Servo 5  Torque") -> ("Signals Out"=w1228:dynamicdata)  [unwired: 2 in, 1 out]
      n370 = xnode "Set Dynamic Data Attributes"("Signals In"=w1272, "Signal Name"="Servo 1 Feedback Position") -> ("Signals Out"=w1236:dynamicdata)  [unwired: 2 in, 1 out]
      n371 = xnode "Set Dynamic Data Attributes"("Signals In"=w1254, "Signal Name"="Servo 3  Torque") -> ("Signals Out"=w1230:dynamicdata)  [unwired: 2 in, 1 out]
      n372 = xnode "Set Dynamic Data Attributes"("Signals In"=w1266, "Signal Name"="Servo 1 Feedback Position") -> ("Signals Out"=w1233:dynamicdata)  [unwired: 2 in, 1 out]
      n373 = xnode "Set Dynamic Data Attributes"("Signals In"=w1256, "Signal Name"="Servo 2  Torque") -> ("Signals Out"=w1231:dynamicdata)  [unwired: 2 in, 1 out]
      n374 = xnode "Set Dynamic Data Attributes"("Signals In"=w1258, "Signal Name"="Servo 1  Torque") -> ("Signals Out"=w1232:dynamicdata)  [unwired: 2 in, 1 out]
      n375 = Merge Signals(w1245, w1244, w1243, w1242, w1241, w1240, w1239, w1238, w1237, w1236, w1235, w1234, w1233, w1232, w1231, w1230, w1229, w1228) -> (w1227:dynamicdata)
      n376 = call "Write To Measurement File"("Signals"=w1227, "Filename"="Filename", "Comment"="Comment") -> ()  [unwired: 14 in, 3 out]
    }
  }
